vi "MoD Main-Optimize - HPLCv2 - Simulate.vi"() -> ()   [LabVIEW 2015]
uses:
  <vilib>/silver_ctls/ArrayMatrixCluster/Real Matrix NI_Silver.ctl
  <vilib>/addons/control/pid/pid.llb/PID Control Input Filter (DBL).vi
  <vilib>/addons/control/pid/autopid.llb/PID Online Autotuning (Relay Feedback).vi
  <vilib>/Analysis/Matrix/Numeric/Conversions/Array To Matrix - RA2.vi
  <vilib>/addons/control/pid/NI_PID_autopid.lvlib
  <vilib>/addons/control/pid/NI_PID_pid.lvlib
  <vilib>/Analysis/Matrix/NI_Matrix.lvlib
panel:
  out "running?":bool=TRUE
  out "new_reactor_volume":bool[](array[boolean])
  out "new_reactor_length":bool[](array[boolean])
  out "Phase_Sensor_voltage":dbl
  out "P_tot":dbl
  out "pause for ms":bool=TRUE
  out "stop_xl_write":bool=TRUE
  out "Num_exp_till_pause":i32
  out "Syringe_pump?":bool=TRUE
  out "System Error":bool=TRUE
  out "error out":errorcluster
  out "Pump setpoint(ul/min) 6":dbl format="%#_13g"
  out "Pump setpoint(ul/min) 5":dbl format="%#_13g"
  out "Pump setpoint(ul/min) 4":dbl format="%#_13g"
  out "Pump setpoint(ul/min) 3":dbl format="%#_13g"
  out "Pump setpoint(ul/min) 2":dbl format="%#_13g"
  out "Pump setpoint(ul/min) 1":dbl format="%#_13g"
  out "Volume (ul) 5":dbl format="%#_13g"
  out "Volume (ul) 4":dbl format="%#_13g"
  out "Volume (ul) 3":dbl format="%#_13g"
  out "Volume (ul) 2":dbl format="%#_13g"
  out "Volume (ul) 1":dbl format="%#_13g"
  in  "tau 5":dbl format="%#_13g"
  out "tau 4":dbl format="%#_13g"
  out "tau 3":dbl format="%#_13g"
  out "tau 2":dbl format="%#_13g"
  out "tau 1":dbl format="%#_13g"
  out "Reactor Length":dbl format="%#_13g"
  out "Flowrate Sensor 2":dbl format="%#_13g"
  out "Flowrate Sensor 1":dbl format="%#_13g"
  out "Pressure 2":dbl format="%#_13g"
  out "Pressure 1":dbl format="%#_13g"
  out "Temperature Control 5":bool=TRUE
  out "Temperature Control 4":bool=TRUE
  out "Temperature Control 3":bool=TRUE
  out "Temperature Control 2":bool=TRUE
  out "Temperature Control 1":bool=TRUE
  out "Temperature SP 5":dbl format="%#_g'C"
  out "Temperature SP 4":dbl format="%#_g'C"
  out "Temperature SP 3":dbl format="%#_g'C"
  out "Temperature SP 2":dbl format="%#_g'C"
  out "Temperature SP 1":dbl format="%#_g'C"
  in  "Bay Temperature 5":dbl
  in  "SSR Duration 5":dbl
  in  "SSR Duration 4":dbl
  in  "SSR Duration 3":dbl
  in  "SSR Duration 2":dbl
  in  "SSR Duration 1":dbl
  in  "Total Product Amount":dbl=1.0 format="%#_gml"
  out "Setup Error":bool=TRUE
  out "Error Message":string
  out "ID CTR":i32
  in  "Tab Control":T1(tab)
  out "Reagent pic 5":picture
  in  "reagent name 5":string
  out "Reagent Pic 4":picture
  in  "reagent name 4":string="octane"
  out "Reagent Pic 3":picture
  in  "reagent  name 3":string="methane"
  in  "Product name":string="benzoic acid"
  in  "reagent name 1":string="hexanedione"
  out "Reagent Pic 1":picture
  in  "Vr5":dbl format="%#_guL"
  in  "Vr4":dbl format="%#_guL"
  in  "Vr3":dbl format="%#_guL"
  in  "Vr2":dbl format="%#_guL"
  in  "Vr1":dbl format="%#_guL"
  in  "System decide help Button":bool
  in  "Reaction Scheme Confirm":bool
  in  "Synthesis Route Array":string[][](array[string])=[["hexanedione", ".5", "PhB(OH)2", "", "", ""], ["ethanol", ".5", "-", "-", "-", "-"], ["methane", ".1", "-", "-", "-", "-"], ["octane", ".1", "-", "-", "-", "-"]]
  in  "System decide help Button 2":bool
  out "Setup Confirm":bool=TRUE
  in  "BAY 1":u16(ring) items=["               Bypass", "         Heated Reactor", "    Small Heated Reator", "         Cooled Reactor", "      Packed Bed Reactor", "          Photo Reactor", "             Separator"]
  in  "BAY 5":u16(ring) items=["               Bypass", "         Heated Reactor", "    Small Heated Reactor", "         Cooled Reactor", "     Packed Bed Reactor", "         Photo Reactor", "             Separator"]
  in  "BAY 4":u16(ring)=1 items=["                Bypass", "         Heated Reactor", "    Small Heated Reactor", "         Cooled Reactor", "     Packed Bed Reactor", "         Photo Reactor", "             Separator"]
  in  "BAY 3":u16(ring) items=["               Bypass", "         Heated Reactor", "    Small Heated Reactor", "         Cooled Reactor", "     Packed Bed Reactor", "          Photo Reactor", "             Separator"]
  in  "BAY 2":u16(ring)=1 items=["               Bypass", "         Heated Reactor", "    Small Heated Reactor", "         Cooled Reactor", "      Packed Bed Reactor", "          Photo Reactor", "             Separator"]
  out "Reagent Pic 2":picture
  out "Product Pic":picture
  in  "reagent name 2":string="ethanol"
  in  "reagent name 6":string
  out "Reagent Pic 6":picture
  in  "System Parameters Help Button":bool
  out "Setup Confirm 2":bool
  in  "System Parameters Confirm Button":bool
  in  "Bay Parameters":T2={"Bay 1 "={"Pump 1 Flowrate"=0.0, "optimize_temp"=FALSE, "optimize_tau"=FALSE, "Run at set flowrate"=FALSE, "Pump 2 Flowrate"=0.0, "Temperature Params"=[40.0, 100.0, 100.0], "pump params 1"=[32.0, 325.0, 325.0], "pump params 2"=[32.0, 325.0, 325.0], "Temperature"=0.0, "Run at set temperature"=FALSE}, "Bay 2 "={"Pump 3 Flowrate"=0.0, "optimize_temp"=TRUE, "optimize_tau"=TRUE, "Run at set flowrate"=FALSE, "Temperature Params"=[40.0, 100.0, 100.0], "Resisdence time params"=[65.0, 650.0, 650.0], "pump_at_ratio"=FALSE, "pump_num_ratio"=0.0, "Temperature"=0.0, "Run at set temperature"=FALSE}, "Bay 3 "={"Pump 4 Flowrate"=100.0, "optimize_temp"=FALSE, "optimize_tau"=FALSE, "Run at set flowrate"=TRUE, "Temperature Params"=[40.0, 100.0, 100.0], "Resisdence time params"=[0.0, 0.0, 0.0], "pump_at_ratio"=FALSE, "pump_num_ratio"=0.0, "Temperature "=0.0, "Run at set temperature"=FALSE}, "Bay 4 "={"Pump 5 Flowrate"=40.0, "Run at set flowrate"=FALSE, "optimize_temp"=TRUE, "optimize_tau"=FALSE, "Resisdence time params"=[0.0, 36.0, 225.0], "Temperature Params"=[40.0, 80.0, 80.0], "pump_at_ratio"=FALSE, "pump_num_ratio"=0.0, "Temperature"=0.0, "Run at set temperature"=FALSE}, "Bay 5 "={"Pump 6 Flowrate"=0.0, "Run at set flowrate"=FALSE, "optimize_temp"=FALSE, "optimize_tau"=FALSE, "Resisdence time params"=[0.0, 0.0, 0.0], "Temperature Params"=[0.0, 0.0, 0.0], "pump_at_ratio"=FALSE, "pump_num_ratio"=0.2, "Temperature"=0.0, "Run at set temperature"=FALSE}, "Excel File Name"="C:\\Users\\Admin\\Dropbox (MIT)\\MoD Files\\Data\\simulations", "hplc File Name"="C:\\Users\\Admin\\Documents\\Data\\HPLC", "Matlab File"="C:\\Users\\Admin\\Dropbox (MIT)\\MoD Files\\Data\\simulation", "Syringe for Pump 2?"=FALSE, "Num_conditons_per_wait"=1.0, "Continue from previous optimization?"=FALSE, "Total Number of Experiments 2"=33.0, "Hplc Wait time(min)"=9.2, "increas_decrease_hplc_peak"=FALSE, "Internal Standard?"=FALSE, "ISTD start"=0.0, "ISTD end"=0.0, "hplc_start"=2.0, "hplc_end"=5.0, "throughput_yield"=FALSE} {"Hplc Wait time(min)" format="%#_13g"; "Bay 5"."Temperature Params" format="%#_g'C"; "Bay 4"."Temperature Params" format="%#_g'C"; "Bay 3"."Temperature Params" format="%#_g'C"; "Bay 2"."Temperature Params" format="%#_g'C"; "Bay 1"."Temperature Params" format="%#_g'C"}
  out "System Confirm Not Clicked":string
  out "best_exp_num":dbl=1.0
  out "temperature_best":dbl[](array[numeric])
  out "Flowrates(ul/min)_best":dbl[](array[numeric])
  out "System Status":u16(ring)=2 caption="Sy" items=["System  Error", "System Running", "System Standby"]
  out "Current Experiment":dbl=1.0
  out "Total Number of Experiments":dbl=33.0
  out "Phase Sensor Chart":T3(graph)
  out "HPLC Analysis":bool
  out "Equlibrating Temperature":bool
  out "Flushing System":bool
  out "Calculate condition":bool
  out "Temperature 5":dbl format="%#_g'C"
  out "Temperature 4":dbl format="%#_g'C"
  out "Temperature 3":dbl format="%#_g'C"
  out "Temperature 2":dbl format="%#_g'C"
  out "Temperature 1":dbl format="%#_g'C"
  out "Flowrate Chart":T4(graph)
  out "Teperature Chart":T5(graph)
  out "Pump Setpoints Chart":T5(graph)
  out "Pressure Chart":T5(graph)
  out "Optimization_loop_index":i32
  out "curr_wait_time":dbl
  out "total_flush_time":dbl
  out "Temp SS? 5":bool=TRUE
  out "Temp SS? 4":bool=TRUE
  out "Temp SS? 3":bool=TRUE
  out "Temp SS? 2":bool=TRUE
  out "Temp SS? 1":bool=TRUE
  out "System Flushed?":bool
  out "stop_button clicked":bool
  out "experiment history":T6
  in  "Number of System Flushes per condtion":dbl
  in  "calculate volume 3":bool
  in  "calculate volume 2":bool
  in  "calculate volume 1":bool
  in  "calculate volume 4":bool
  in  "calculate volume 5":bool
  in  "Extra system dead volume":dbl format="%#_gul"
  in  "new reactor length? 1":bool
  in  "tube_length(in)":dbl[](array[numeric])=[188.0, 188.0, 10.0, 10.0, 10.0]
  out "Pause Before Analysis":bool
  out "Chiller COMM Port":bool
  out "Arduino COMM Port 2":bool
  out "Temperature Sensor COMM Port":bool
  out "Flow Rate":bool
  out "Pressure":bool
  out "Pump COMM Port":bool
  in  "COMM Port :: Milligat Pumps":refnum<visa-resource-name>="COM10"
  in  "Arduino COMM Port":refnum<visa-resource-name>="COM3"
  in  "Sample Valve COMM::Port":refnum<visa-resource-name>="COM6"
  in  "COMM Port:: Harvard Syringe Pump":refnum<visa-resource-name>="COM5"
  in  "tube_id(in)":enum16{".01", ".02", ".03", ".04"}[](array[ring])=[enum.".02", enum.".03", enum.".03", enum.".03", enum.".03"]
  out "Total System Resisdence Time(min)":dbl
  in  "Debug_run_button":bool
  in  "new reactor length? 2":bool
  in  "new reactor length? 3":bool
  in  "new reactor length? 4":bool
  in  "new reactor length? 5":bool
  out "Stop":bool=TRUE
  in  "Run_Stop_cluster":T7
  # "Molecules on Demand"
  # "Synthetic Route"
  # "5"
  # "6"
  # "4"
  # "Product"
  # "1"
  # "2"
  # "3"
  # "Reagent List"
  # "Concentration(M)"
  # "Molecule"
  # "1"
  # "1"
  # "2"
  # "2"
  # "3"
  # "3"
  # "4"
  # "4"
  # "5"
  # "6"
  # "5"
  # "6"
  # "Product"
  # "Reactor Volume:"
  # "Optimization Parameters"
  # "Pause after"
  # "Experiments"
  # "Optimize for"
  # "to"
  # "of HPLC Peak from"
  # "from"
  # "to"
  # "min"
  # "min"
  # "HPLC runtime"
  # "# Iterations"
  # "Reporting"
  # "Excel Output File Name"
  # "HPLC File Path"
  # "MATLAB File Path"
  # "Temperature"
  # "Flowrate(ul/min)"
  # "Lower Bound"
  # "Upper Bound"
  # "Optimize?"
  # "-or-"
  # "Run at"
  # "times incoming flow"
  # "Setpoint"
  # "Temperature"
  # "Flowrate(ul/min)"
  # "Lower Bound"
  # "Upper Bound"
  # "Optimize?"
  # "-or-"
  # "Run at"
  # "times incoming flow"
  # "Setpoint"
  # "Temperature"
  # "Flowrate(ul/min)"
  # "Lower Bound"
  # "Upper Bound"
  # "Optimize?"
  # "-or-"
  # "Run at"
  # "times incoming flow"
  # "Setpoint"
  # "Temperature"
  # "Flowrate 3 (ul/min)"
  # "Lower Bound"
  # "Upper Bound"
  # "Optimize?"
  # "-or-"
  # "Run at"
  # "times incoming flow"
  # "Setpoint"
  # "Temperature"
  # "Flowrate 1(ul/min)"
  # "Flowrate 2(ul/min)"
  # "Lower Bound"
  # "Upper Bound"
  # "Optimize?"
  # "Setpoint"
  # "Pressure (psi)"
  # "System Status"
  # "Temperature('C)"
  # "BAY"
  # "1"
  # "2"
  # "3"
  # "4"
  # "5"
  # "Pump Flowrate Setpoint(ul/min)"
  # "Flowrate (ul/min)"
  # "Phase Sensor"
  # "Current Experiment"
  # "Temperature('C)"
  # "Flowrate(ul/min)"
  # "Exp"
  # "Current Best Condition"
  # "Time to reach steady state:"
  # "Current Wait Time:"
  # "Experimental Steps"
  # "Calculated new conditions"
  # "Flushed System"
  # "Analyzed HPLC"
  # "Equilibrated Temperature"
  # "Tube Length (cm)"
  # "Bay"
  # "Tube ID (in)"
  # "Calculate Volume"
  # "Use new tube length"
  # "1."
  # "2."
  # "3."
  # "4."
  # "5."
  # "Reactor Lengths\n*Heated Reactor - 188cm * Small Reactor - 99cm * Bypass - 10cm * Separator - *"
  # "All Experimental Data"
  # "P1"
  # "P2"
  # "P3"
  # "P4"
  # "P5"
  # "P6"
  # "T1"
  # "T2"
  # "T3"
  # "T4"
  # "T5"
  # "Obj_fun"
  # "HPLC_Data"
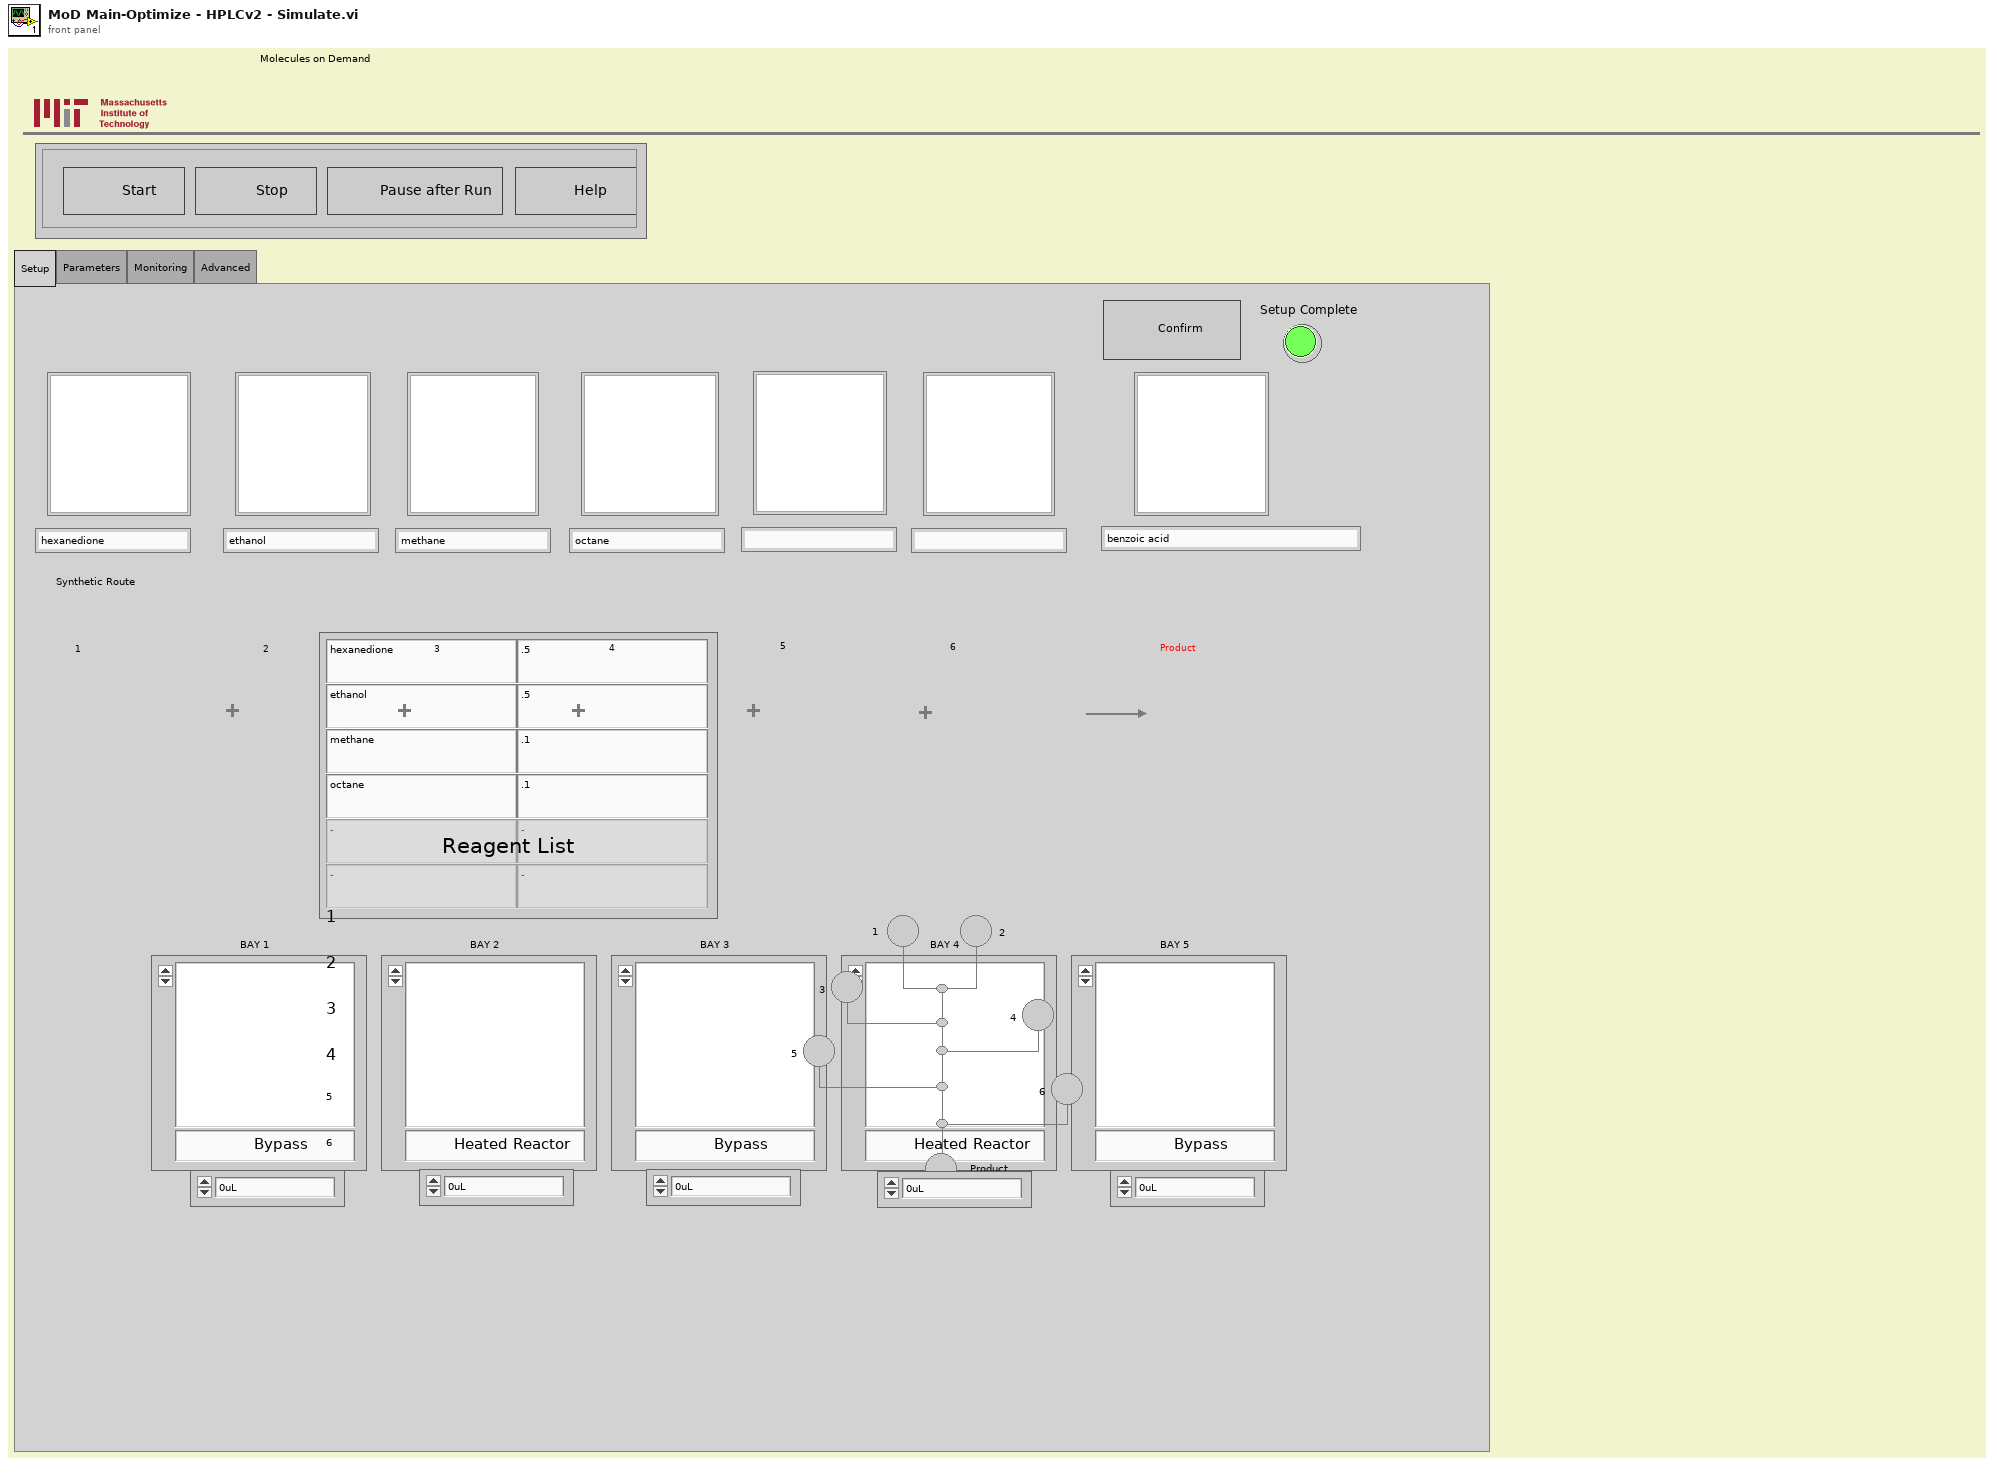
[diagram p1: front panel]
types:
  T1 = enum32{"Setup", "Parameters", "Monitoring", "Advanced"}
  T2 = cluster{"Bay 1 ":cluster{"Pump 1 Flowrate":dbl, "optimize_temp":bool, "optimize_tau":bool, "Run at set flowrate":bool, "Pump 2 Flowrate":dbl, "Temperature Params":dbl[], "pump params 1":dbl[], "pump params 2":dbl[], "Temperature":dbl, "Run at set temperature":bool}, "Bay 2 ":cluster{"Pump 3 Flowrate":dbl, "optimize_temp":bool, "optimize_tau":bool, "Run at set flowrate":bool, "Temperature Params":dbl[], "Resisdence time params":dbl[], "pump_at_ratio":bool, "pump_num_ratio":dbl, "Temperature":dbl, "Run at set temperature":bool}, "Bay 3 ":cluster{"Pump 4 Flowrate":dbl, "optimize_temp":bool, "optimize_tau":bool, "Run at set flowrate":bool, "Temperature Params":dbl[], "Resisdence time params":dbl[], "pump_at_ratio":bool, "pump_num_ratio":dbl, "Temperature ":dbl, "Run at set temperature":bool}, "Bay 4 ":cluster{"Pump 5 Flowrate":dbl, "Run at set flowrate":bool, "optimize_temp":bool, "optimize_tau":bool, "Resisdence time params":dbl[], "Temperature Params":dbl[], "pump_at_ratio":bool, "pump_num_ratio":dbl, "Temperature":dbl, "Run at set temperature":bool}, "Bay 5 ":cluster{"Pump 6 Flowrate":dbl, "Run at set flowrate":bool, "optimize_temp":bool, "optimize_tau":bool, "Resisdence time params":dbl[], "Temperature Params":dbl[], "pump_at_ratio":bool, "pump_num_ratio":dbl, "Temperature":dbl, "Run at set temperature":bool}, "Excel File Name":string, "hplc File Name":string, "Matlab File":string, "Syringe for Pump 2?":bool, "Num_conditons_per_wait":dbl, "Continue from previous optimization?":bool, "Total Number of Experiments 2":dbl, "Hplc Wait time(min)":dbl, "increas_decrease_hplc_peak":bool, "Internal Standard?":bool, "ISTD start":dbl, "ISTD end":dbl, "hplc_start":dbl, "hplc_end":dbl, "throughput_yield":bool}
  T3 = cluster{"[0]":u8, "[1]":u8, "[2]":u8, "[3]":u8, "[4]":u8, "[5]":u8, "[6]":u8, "[7]":u8, "[8]":u8}
  T4 = cluster{"[0]":i32, "[1]":i32, "[2]":i32, "[3]":i32, "[4]":i32, "[5]":i32, "[6]":i32, "[7]":i32, "[8]":i32}
  T5 = cluster{"[0]":dbl, "[1]":dbl, "[2]":dbl, "[3]":dbl, "[4]":dbl, "[5]":dbl, "[6]":dbl, "[7]":dbl, "[8]":dbl}
  T6 = typedef "Real Matrix NI_Silver.ctl" = dbl[][]
  T7 = cluster{"Stop":bool, "Run":bool, "Stop Run Button":bool, "Help Button":bool}
  T8 = cluster{"Proportional gain Kc":dbl, "Integral time Ti (sec)":dbl, "Derivative time Ti (sec)":dbl}
  T9 = cluster{"type of controller":enum16{"P", "PI", "PID"}, "relay cycles":i32, "relay amplitude":dbl, "control specifications":enum16{"Fast", "Normal", "Slow"}, "PV noise level":dbl}
  T10 = typedef "imagedata.ctl" = cluster{"image type":i32, "image depth":i32, "image":u8[], "mask":u8[], "colors":u32[], "Rectangle":cluster{"left":i16, "top":i16, "right":i16, "bottom":i16}}
  T11 = cluster{"proportional gain (Kc)":dbl, "integral time (Ti, min)":dbl, "derivative time (Td, min)":dbl}
  T12 = enum16{"Left Button", "Center Button", "Right Button", "Window Close"}
  T13 = typedef "NI_Matrix.lvlib/RealMatrix.ctl" = dbl[][]
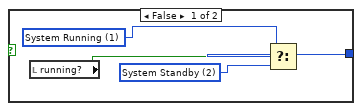
[diagram p4: hidden frame]
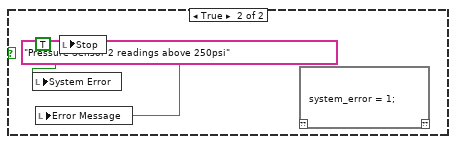
[diagram p5: hidden frame]
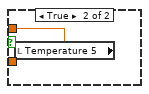
[diagram p7: hidden frame]
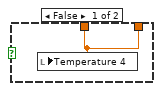
[diagram p8: hidden frame]
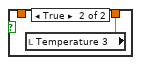
[diagram p9: hidden frame]
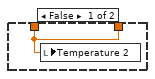
[diagram p10: hidden frame]
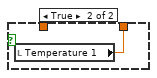
[diagram p11: hidden frame]
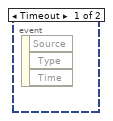
[diagram p12: hidden frame]
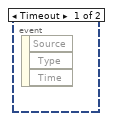
[diagram p14: hidden frame]
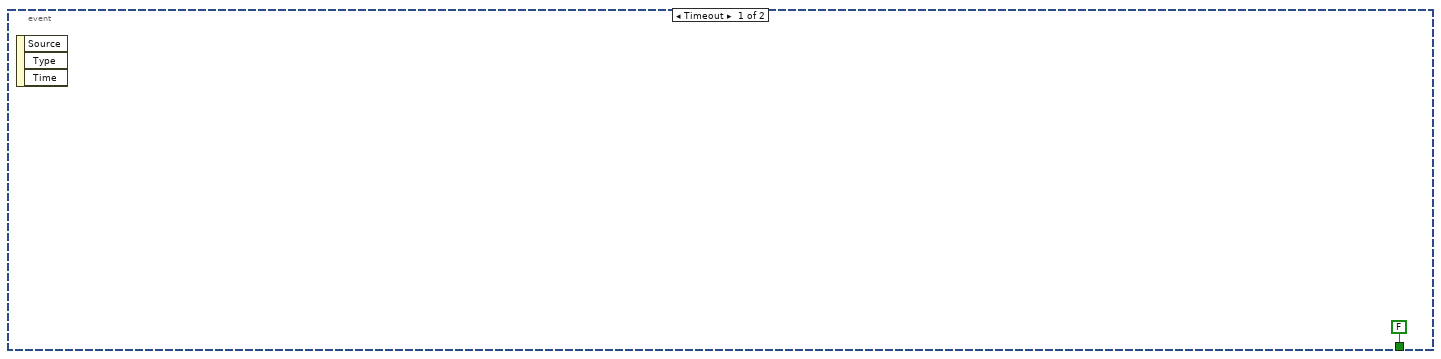
[diagram p17: hidden frame]
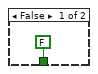
[diagram p18: hidden frame]
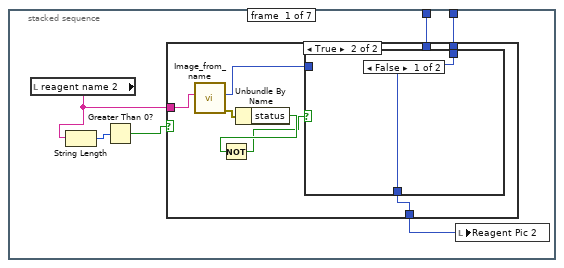
[diagram p19: hidden frame]
diagram:
  # "Assume User always uses the first bay first"
  n1 = flat-sequence {
    tunnel: ["COMM Port :: Milligat Pumps"] -> w6
    tunnel: ["Arduino COMM Port"] -> w5
    tunnel: ["COMM Port:: Harvard Syringe Pump"] -> w2
    tunnel: ["Bay Parameters"] -> w1
    tunnel: [w54] -> w7
    tunnel: w6 -> [w54]
    tunnel: w5 -> [_]
    tunnel: [w48] -> w4
    tunnel: [w46] -> w3
    tunnel: w2 -> [w46]
    tunnel: w1 -> [w44]
    tunnel: w7 -> [w58]
    tunnel: w4 -> [w57]
    tunnel: w3 -> [w55]
    frame #0 {
      w32 = FALSE ("Equlibrating Temperature")
      n2 = disable-structure shown="Disabled" {
        frame Disabled {
          # "IR Sensor"
        }
        frame Enabled {
        }
      }
      n3 = script code="TempArr1=[23 23 23 23 23 23 23 23 23 23]';\nTempArr2=[23 23 23 23 23 23 23 23 23 23]';\nTempArr3=[23 23 23 23 23 23 23 23 23 23]';\nTempArr4=[23 23 23 23 23 23 23 23 23 23]';\nTempArr5=[23 23 23 23 23 23 23 23 23 23]';\ntemp_error1 =0;\ntemp_error2 =0;\ntemp_error3 =0;\ntemp_error4 =0;\ntemp_error5 =0;\ntemp_check1 = 0;\ntemp_check2 = 0;\ntemp_check3 = 0;\ntemp_check4 = 0;\ntemp_check5 = 0;\nT1=23;\nT2=23;\nT3=23;\nT4=23;\nT5=23;"() -> ()  [unwired: 1 in, 1 out]
      n4 = Build Array("calculate volume 1", "calculate volume 2", "calculate volume 3", "calculate volume 4", "calculate volume 5") -> (→"new_reactor_volume":bool[])
      n5 = Build Array("new reactor length? 1", "new reactor length? 2", "new reactor length? 3", "new reactor length? 4", "new reactor length? 5") -> (→"new_reactor_length":bool[])
      "Stop" <- FALSE ("Stop")
      "ID CTR" <- 0
      "Setup Confirm" <- FALSE ("Setup Confirm")
      "Error Message" <- "System shutdown sucessfully. No errors to report." ("Error Message")
      "Setup Error" <- FALSE ("Setup Error")
      "Reactor Length" <- 10.5
      "System Error" <- FALSE ("System Error")
      "Num_exp_till_pause" <- 0 ("Num_exp_till_pause")
      "Equlibrating Temperature" <- w32
      "Calculate condition" <- w32
      "Flushing System" <- w32
      "HPLC Analysis" <- w32
      "stop_xl_write" <- FALSE ("stop_xl_write")
      "Pump setpoint(ul/min) 1" <- 0.0 ("Pump setpoint(ul/min) 1")
      "Pump setpoint(ul/min) 2" <- 0.0 ("Pump setpoint(ul/min) 2")
      "Pump setpoint(ul/min) 4" <- 0.0 ("Pump setpoint(ul/min) 4")
      "Pump setpoint(ul/min) 6" <- 0.0 ("Pump setpoint(ul/min) 6")
      "Pump setpoint(ul/min) 3" <- 0.0 ("Pump setpoint(ul/min) 3")
      "Pump setpoint(ul/min) 5" <- 0.0 ("Pump setpoint(ul/min) 5")
      "pause for ms" <- FALSE ("pause for ms")
      "Setup Confirm 2" <- FALSE ("Setup Confirm 2")
      "running?" <- FALSE ("running?")
    }
    frame #1 {
      w43 = FALSE
      w53 = 23
      (unwired) path "C:/Users/User1/Documents/Lab/MoD/Images"
      n6 = disable-structure shown="Disabled" {
        frame Disabled {
          n7 = local read "BAY 2"() -> ()  [unwired: 1 out]
          n8 = local read "BAY 3"() -> ()  [unwired: 1 out]
          n9 = local read "BAY 4"() -> ()  [unwired: 1 out]
          n10 = local read "BAY 5"() -> ()  [unwired: 1 out]
          n11 = local read "BAY 1"() -> ()  [unwired: 1 out]
        }
        frame Enabled {
        }
      }
      n12 = local write "Debug_run_button"(TRUE) -> ()
      n13 = local write "System Parameters Confirm Button"(w43) -> ()
      n14 = local write "Setup Confirm 2"(w43) -> ()
      n15 = Unbundle By Name(w44) -> ("Syringe for Pump 2?"=→"Syringe_pump?":bool)
      n16 = local write "Temperature 1"(w53) -> ()
      n17 = local write "Temperature 2"(w53) -> ()
      n18 = local write "Temperature 3"(w53) -> ()
      n19 = local write "Temperature 4"(w53) -> ()
      n20 = local write "Temperature 5"(w53) -> ()
      n21 = local write "Temperature SP 1"(w53) -> ()
      n22 = local write "Temperature SP 2"(w53) -> ()
      n23 = local write "Temperature SP 3"(w53) -> ()
      n24 = local write "Temperature SP 4"(w53) -> ()
      n25 = local write "Temperature SP 5"(w53) -> ()
      n26 = Current VI's Path() -> (path=w52:path)
      n27 = Strip Path(path=w52) -> (stripped path=w50:path)  [unwired: 1 out]
      n28 = Strip Path(path=w50) -> (stripped path=w49:path)  [unwired: 1 out]
      n29 = Build Path(base path=w49, name or relative path="MATLAB") -> (appended path=w48:path)
    }
    frame #2 {
      # "Main Help Dialog Popup"
      n30 = while {
        stop <- w1172 stop-if-true
        n31 = event shown="[6] \"Run_Stop_cluster.Run\": Value Change" {
          selector: _ -> [_ _ _ _ _ _ _]
          dyn-events: _ -> [_ _ _ _ _ _ _]
          timeout: 100 -> [_ _ _ _ _ _ _]
          event Timeout {
            n32 = event-data() -> ()  [unwired: 1 in, 3 out]
          }
          event "Run_Stop_cluster.Help Button": Value Change {
            n33 = local read "Run_Stop_cluster"() -> (w1175:T7)
            n34 = event-data() -> ()  [unwired: 1 in, 4 out]
            n35 = Unbundle By Name(w1175) -> ("Help Button"=w1174:bool)
            n36 = case shown="True" w1174 {
              frame False {
              }
              frame True {
                n37 = call "help.vi"() -> ()  [unwired: 11 in]
              }
            }
          }
          event "System decide help Button": Value Change {
            n38 = event-data() -> ()  [unwired: 1 in, 5 out]
            n39 = call "help_synthesis_man-auto_instructions.vi"() -> ()  [unwired: 12 in]
          }
          event "System Parameters Help Button": Value Change {
            n40 = event-data() -> ()  [unwired: 1 in, 5 out]
            n41 = call "help_parameters_setup.vi"() -> ()  [unwired: 12 in]
          }
          event "System decide help Button 2": Value Change {
            n42 = event-data() -> ()  [unwired: 1 in, 5 out]
            n43 = call "help_synthesis_route_instructions.vi"() -> ()  [unwired: 12 in]
          }
          event "Run_Stop_cluster.Stop": Value Change {
            n44 = event-data() -> ()  [unwired: 1 in, 5 out]
            n45 = local write "Stop"(TRUE) -> ()
          }
          event "Run_Stop_cluster.Run": Value Change {
            n46 = event-data() -> ()  [unwired: 1 in, 5 out]
            n47 = local write "running?"(TRUE) -> ()
          }
        }
        n48 = local read "Stop"() -> (w1172:bool)
      }
      n49 = stacked-sequence {
        tunnel: w58 -> [_ _ _ _]
        tunnel: w57 -> [_ w364 _ _]
        tunnel: w55 -> [_ _ _ w526]
        frame #0 {
          # "System Setup"
          n50 = while {
            stop <- w160 stop-if-true
            n51 = event shown="[1] \"Reaction Scheme Confirm\": Value Change" {
              selector: _ -> [_ _]
              dyn-events: _ -> [_ _]
              timeout: 400 -> [_ _]
              tunnel: [FALSE w180] -> w162
              event Timeout {
                n52 = event-data() -> ()  [unwired: 1 in, 3 out]
              }
              event "Reaction Scheme Confirm": Value Change {
                n53 = event-data() -> ()  [unwired: 1 in, 6 out]
                n54 = local read "Reaction Scheme Confirm"() -> (w184:bool)
                n55 = local read "Setup Confirm"() -> (w182:bool)
                n56 = Not(x=w182) -> (.not. x?=w181:bool)
                n57 = And(x=w184, y=w181) -> (x .and. y?=w183:bool)
                n58 = case shown="True" w183 {
                  tunnel: [FALSE w186] -> w180
                  frame False {
                  }
                  frame True {
                    n59 = flat-sequence {
                      tunnel: [w354] -> w186
                      frame #0 {
                        n60 = local write "Setup Error"(FALSE) -> ()
                      }
                      frame #1 {
                        n61 = local read "Synthesis Route Array"() -> (w190:string[][])
                        n62 = Index Array(array=w190, index (col)=0 ("disabled index (col)")) -> (element=w188:string[])  [unwired: 1 in]
                        n63 = Array Size(array=w188) -> (size(s)=w191:i32)
                        n64 = script code="MATLAB script"("reagentNum"=w191) -> ()  [unwired: 1 in, 1 out]
                      }
                      frame #2 {
                        w194 = "C:\\Users\\HPLC\\Dropbox (MIT)\\MoD Files\\LabVIEW\\Mod 2014\\MoD Main Folder\\Chemical Image\\" ("string")
                        n65 = String To Path(string=w194) -> (path=w200:path)
                        n66 = Build Path(base path=w200, name or relative path="image_not_found3.jpg") -> (appended path=w199:path)
                        n67 = String To Path(string=w194) -> (path=w197:path)
                        n68 = call <vilib>:"Read JPEG File.vi"("path to JPEG file"=w199) -> ("image data"=w202:T10)  [unwired: 1 in, 9 out]
                        n69 = Build Path(base path=w197, name or relative path="blank image.jpg") -> (appended path=w195:path)
                        n70 = call <vilib>:"Read JPEG File.vi"("path to JPEG file"=w195) -> ("image data"=w198:T10)  [unwired: 1 in, 9 out]
                        n71 = call <vilib>:"Draw Flattened Pixmap.vi"("image data"=w202) -> ("new picture"=w193:picture)  [unwired: 3 in, 5 out]
                        n72 = call <vilib>:"Draw Flattened Pixmap.vi"("image data"=w198) -> ("new picture"=w192:picture)  [unwired: 3 in, 5 out]
                        n73 = stacked-sequence {
                          tunnel: w193 -> [w208 w225 w242 w259 w276 w290 w307]
                          tunnel: w192 -> [w206 w223 w240 w257 w274 w291 w308]
                          frame #0 {
                            n74 = local read "reagent name 2"() -> (w204:string)
                            n75 = String Length(string=w204) -> (length=w207:i32)
                            n76 = Greater Than 0?(x=w207) -> (x > 0?=w205:bool)
                            n77 = case shown="True" w205 {
                              tunnel: w208 -> [_ w214]
                              tunnel: w206 -> [w209 _]
                              tunnel: [w209 w213] -> w203
                              tunnel: w204 -> [_ w212]
                              frame False {
                              }
                              frame True {
                                n78 = call "Image_from_name.vi"("Chemical Name"=w212) -> ("error out"=w215:errorcluster, "Downloaded Picture"=w216:picture)  [unwired: 8 in, 1 out]
                                n79 = Unbundle By Name(w215) -> ("status"=w211:bool)
                                n80 = Not(x=w211) -> (.not. x?=w210:bool)
                                n81 = case shown="False" w210 {
                                tunnel: w216 -> [_ w219]
                                tunnel: [w217 w218] -> w213
                                tunnel: w214 -> [w217 _]
                                frame False {
                                }
                                frame True {
                                n82 = call <vilib>:"Draw Flattened Pixmap.vi"("picture"=w219) -> ("new picture"=w218:picture)  [unwired: 8 in]
                                }
                                }
                              }
                            }
                            n83 = local write "Reagent Pic 2"(w203) -> ()
                          }
                          frame #1 {
                            n84 = local read "reagent name 1"() -> (w220:string)
                            n85 = String Length(string=w220) -> (length=w224:i32)
                            n86 = Greater Than 0?(x=w224) -> (x > 0?=w222:bool)
                            n87 = case shown="True" w222 {
                              tunnel: w225 -> [_ w231]
                              tunnel: w223 -> [w226 _]
                              tunnel: [w226 w230] -> w221
                              tunnel: w220 -> [_ w229]
                              frame False {
                              }
                              frame True {
                                n88 = call "Image_from_name.vi"("Chemical Name"=w229) -> ("error out"=w232:errorcluster, "Downloaded Picture"=w233:picture)  [unwired: 8 in, 1 out]
                                n89 = Unbundle By Name(w232) -> ("status"=w228:bool)
                                n90 = Not(x=w228) -> (.not. x?=w227:bool)
                                n91 = case shown="True" w227 {
                                tunnel: w233 -> [_ w236]
                                tunnel: [w234 w235] -> w230
                                tunnel: w231 -> [w234 _]
                                frame False {
                                }
                                frame True {
                                n92 = call <vilib>:"Draw Flattened Pixmap.vi"("picture"=w236) -> ("new picture"=w235:picture)  [unwired: 8 in]
                                }
                                }
                              }
                            }
                            n93 = local write "Reagent Pic 1"(w221) -> ()
                          }
                          frame #2 {
                            n94 = local read "Product name"() -> (w237:string)
                            n95 = String Length(string=w237) -> (length=w241:i32)
                            n96 = Greater Than 0?(x=w241) -> (x > 0?=w239:bool)
                            n97 = case shown="True" w239 {
                              tunnel: w242 -> [_ w248]
                              tunnel: w240 -> [w243 _]
                              tunnel: [w243 w247] -> w238
                              tunnel: w237 -> [_ w246]
                              frame False {
                              }
                              frame True {
                                n98 = call "Image_from_name.vi"("Chemical Name"=w246) -> ("error out"=w249:errorcluster, "Downloaded Picture"=w250:picture)  [unwired: 8 in, 1 out]
                                n99 = Unbundle By Name(w249) -> ("status"=w244:bool)
                                n100 = Not(x=w244) -> (.not. x?=w245:bool)
                                n101 = case shown="False" w245 {
                                tunnel: w250 -> [_ w253]
                                tunnel: [w251 w252] -> w247
                                tunnel: w248 -> [w251 _]
                                frame False {
                                }
                                frame True {
                                n102 = call <vilib>:"Draw Flattened Pixmap.vi"("picture"=w253) -> ("new picture"=w252:picture)  [unwired: 8 in]
                                }
                                }
                              }
                            }
                            n103 = local write "Product Pic"(w238) -> ()
                          }
                          frame #3 {
                            n104 = local read "reagent name 6"() -> (w254:string)
                            n105 = String Length(string=w254) -> (length=w258:i32)
                            n106 = Greater Than 0?(x=w258) -> (x > 0?=w256:bool)
                            n107 = case shown="True" w256 {
                              tunnel: w259 -> [_ w265]
                              tunnel: w257 -> [w260 _]
                              tunnel: [w260 w264] -> w255
                              tunnel: w254 -> [_ w263]
                              frame False {
                              }
                              frame True {
                                n108 = call "Image_from_name.vi"("Chemical Name"=w263) -> ("error out"=w266:errorcluster, "Downloaded Picture"=w267:picture)  [unwired: 8 in, 1 out]
                                n109 = Unbundle By Name(w266) -> ("status"=w261:bool)
                                n110 = Not(x=w261) -> (.not. x?=w262:bool)
                                n111 = case shown="False" w262 {
                                tunnel: w267 -> [_ w270]
                                tunnel: [w268 w269] -> w264
                                tunnel: w265 -> [w268 _]
                                frame False {
                                }
                                frame True {
                                n112 = call <vilib>:"Draw Flattened Pixmap.vi"("picture"=w270) -> ("new picture"=w269:picture)  [unwired: 8 in]
                                }
                                }
                              }
                            }
                            n113 = local write "Reagent Pic 6"(w255) -> ()
                          }
                          frame #4 {
                            n114 = local read "reagent name 5"() -> (w271:string)
                            n115 = String Length(string=w271) -> (length=w275:i32)
                            n116 = Greater Than 0?(x=w275) -> (x > 0?=w273:bool)
                            n117 = case shown="True" w273 {
                              tunnel: w276 -> [_ w282]
                              tunnel: w274 -> [w277 _]
                              tunnel: [w277 w281] -> w272
                              tunnel: w271 -> [_ w280]
                              frame False {
                              }
                              frame True {
                                n118 = call "Image_from_name.vi"("Chemical Name"=w280) -> ("error out"=w283:errorcluster, "Downloaded Picture"=w284:picture)  [unwired: 8 in, 1 out]
                                n119 = Unbundle By Name(w283) -> ("status"=w278:bool)
                                n120 = Not(x=w278) -> (.not. x?=w279:bool)
                                n121 = case shown="False" w279 {
                                tunnel: w284 -> [_ w287]
                                tunnel: [w285 w286] -> w281
                                tunnel: w282 -> [w285 _]
                                frame False {
                                }
                                frame True {
                                n122 = call <vilib>:"Draw Flattened Pixmap.vi"("picture"=w287) -> ("new picture"=w286:picture)  [unwired: 8 in]
                                }
                                }
                              }
                            }
                            n123 = local write "Reagent pic 5"(w272) -> ()
                          }
                          frame #5 {
                            n124 = local read "reagent name 4"() -> (w288:string)
                            n125 = String Length(string=w288) -> (length=w293:i32)
                            n126 = Greater Than 0?(x=w293) -> (x > 0?=w292:bool)
                            n127 = case shown="True" w292 {
                              tunnel: w290 -> [_ w299]
                              tunnel: w291 -> [w294 _]
                              tunnel: [w294 w298] -> w289
                              tunnel: w288 -> [_ w297]
                              frame False {
                              }
                              frame True {
                                n128 = call "Image_from_name.vi"("Chemical Name"=w297) -> ("error out"=w300:errorcluster, "Downloaded Picture"=w301:picture)  [unwired: 8 in, 1 out]
                                n129 = Unbundle By Name(w300) -> ("status"=w295:bool)
                                n130 = Not(x=w295) -> (.not. x?=w296:bool)
                                n131 = case shown="False" w296 {
                                tunnel: w301 -> [_ w304]
                                tunnel: [w302 w303] -> w298
                                tunnel: w299 -> [w302 _]
                                frame False {
                                }
                                frame True {
                                n132 = call <vilib>:"Draw Flattened Pixmap.vi"("picture"=w304) -> ("new picture"=w303:picture)  [unwired: 8 in]
                                }
                                }
                              }
                            }
                            n133 = local write "Reagent Pic 4"(w289) -> ()
                          }
                          frame #6 {
                            n134 = local read "reagent  name 3"() -> (w305:string)
                            n135 = String Length(string=w305) -> (length=w310:i32)
                            n136 = Greater Than 0?(x=w310) -> (x > 0?=w309:bool)
                            n137 = case shown="True" w309 {
                              tunnel: w307 -> [_ w316]
                              tunnel: w308 -> [w311 _]
                              tunnel: [w311 w315] -> w306
                              tunnel: w305 -> [_ w314]
                              frame False {
                              }
                              frame True {
                                n138 = call "Image_from_name.vi"("Chemical Name"=w314) -> ("error out"=w317:errorcluster, "Downloaded Picture"=w318:picture)  [unwired: 8 in, 1 out]
                                n139 = Unbundle By Name(w317) -> ("status"=w312:bool)
                                n140 = Not(x=w312) -> (.not. x?=w313:bool)
                                n141 = case shown="False" w313 {
                                tunnel: w318 -> [_ w321]
                                tunnel: [w319 w320] -> w315
                                tunnel: w316 -> [w319 _]
                                frame False {
                                }
                                frame True {
                                n142 = call <vilib>:"Draw Flattened Pixmap.vi"("picture"=w321) -> ("new picture"=w320:picture)  [unwired: 8 in]
                                }
                                }
                              }
                            }
                            n143 = local write "Reagent Pic 3"(w306) -> ()
                          }
                        }
                      }
                      frame #3 {
                        n144 = local read "BAY 1"() -> (w332:u16)
                        n145 = local read "BAY 2"() -> (w331:u16)
                        n146 = local read "BAY 3"() -> (w330:u16)
                        n147 = local read "BAY 4"() -> (w329:u16)
                        n148 = local read "BAY 5"() -> (w328:u16)
                        n149 = local read "tube_id(in)"() -> (w339:enum16{".01", ".02", ".03", ".04"}[])
                        n150 = local read "Vr4"() -> (w342:dbl)
                        n151 = local read "tube_length(in)"() -> (w340:dbl[])
                        n152 = Build Array(w332, w331, w330, w329, w328) -> (w327:u16[])
                        n153 = local read "Vr3"() -> (w343:dbl)
                        n154 = local read "new_reactor_length"() -> (w337:bool[])
                        n155 = local read "Vr1"() -> (w345:dbl)
                        n156 = local read "Vr5"() -> (w341:dbl)
                        n157 = local read "Vr2"() -> (w344:dbl)
                        n158 = local read "new_reactor_volume"() -> (w335:bool[])
                        n159 = for {
                          N: 5 -> [_]
                          tunnel: w335 -> [w349] mode=indexing
                          tunnel: [w346] -> w333 mode=indexing
                          n160 = Select(t=1.0, s=w349, f=0.0) -> (s? t:f=w346:dbl)
                        }
                        n161 = for {
                          N: 5 -> [_]
                          tunnel: w337 -> [w353] mode=indexing
                          tunnel: [w350] -> w336 mode=indexing
                          n162 = Select(t=1.0, s=w353, f=0.0) -> (s? t:f=w350:dbl)
                        }
                        n163 = script code="tube_diameters = [.01,.02,.03,.04];\naddpath('C:\\Users\\HPLC\\Dropbox (MIT)\\MoD Files\\MATLAB');\ncalculate_reactor_volumes;"("BayConfig"=w327, "Vr1"=w345, "Vr2"=w344, "Vr3"=w343, "Vr4"=w342, "Vr5"=w341, "tube_length"=w340, "tube_id"=w339, "new_len_react"=w336, "new_vol_react"=w333) -> ("Vr1"=w326:dbl, "Vr2"=w325:dbl, "Vr3"=w324:dbl, "Vr4"=w323:dbl, "Vr5"=w322:dbl)  [unwired: 1 in, 1 out]
                        n164 = local write "Vr1"(w326) -> ()
                        n165 = local write "Vr2"(w325) -> ()
                        n166 = local write "Vr3"(w324) -> ()
                        n167 = local write "Vr4"(w323) -> ()
                        n168 = local write "Vr5"(w322) -> ()
                      }
                      frame #4 {
                        n169 = local read "Setup Error"() -> (w356:bool)
                        n170 = case shown="True" w356 {
                          tunnel: [TRUE FALSE] -> w354
                          tunnel: ["" "Sytem setup has not been confirmed!"] -> w355
                          frame False {
                          }
                          frame True {
                            n171 = local read "Error Message"() -> (w361:string)
                            n172 = One Button Dialog(message=w361) -> ()  [unwired: 1 in, 1 out]
                          }
                        }
                        n173 = local write "System Confirm Not Clicked"(w355) -> ()
                        n174 = local write "Setup Confirm"(w354) -> ()
                      }
                    }
                  }
                }
              }
            }
            n175 = local read "Stop"() -> (w161:bool)
            n176 = Or(x=w162, y=w161) -> (x .or. y?=w160:bool)
            n177 = disable-structure shown="Disabled" {
              disable-tunnel: 400 -> [w168 _]
              frame Disabled {
                n178 = event shown="[1]" {
                  selector: _ -> [_ _]
                  dyn-events: _ -> [_ _]
                  timeout: w168 -> [_ _]
                  event Timeout {
                    n179 = event-data() -> ()  [unwired: 1 in, 3 out]
                  }
                  event #1 (no event record) {
                    n180 = event-data() -> ()  [unwired: 1 in, 6 out]
                    n181 = local read "Setup Confirm"() -> (w169:bool)
                    n182 = local read "Reaction Scheme Confirm"() -> (w170:bool)
                    n183 = Not(x=w169) -> (.not. x?=w172:bool)
                    n184 = And(x=w170, y=w172) -> (x .and. y?=w171:bool)
                    n185 = case shown="True" w171 {
                      frame False {
                      }
                      frame True {
                        w174 = u16 0 items=["                     Bypass", "                Hot Reactor", "                 Separator"] ("BAY 5")
                        w175 = u16 0 items=["                     Bypass", "                Hot Reactor", "                  Separator"] ("BAY 4")
                        w176 = u16 0 items=["                     Bypass", "                 Hot Reactor", "                  Separator"] ("BAY 3")
                        w177 = u16 0 items=["                     Bypass", "                Hot Reactor", "                  Separator"] ("BAY 2")
                        w178 = u16 0 items=["                 Bypass", "             Hot Reactor", "               Separator"] ("BAY 1")
                        n186 = local write "BAY 3"(w176) -> ()
                        n187 = local write "BAY 4"(w175) -> ()
                        n188 = local write "BAY 5"(w174) -> ()
                        n189 = local write "BAY 2"(w177) -> ()
                        n190 = local write "BAY 1"(w178) -> ()
                        n191 = local write "Synthesis Route Array"(string[][] [["3-Br-Pyridine _ Biphenyl", "K2CO3", "PhB(OH)2", "", "", ""]] ("Synthesis Route Array")) -> ()
                      }
                    }
                  }
                }
              }
              frame Enabled {
              }
            }
            n192 = disable-structure shown="Disabled" {
              disable-tunnel: 400 -> [w164 _]
              frame Disabled {
                n193 = event shown="[1]" {
                  selector: _ -> [_ _]
                  dyn-events: _ -> [_ _]
                  timeout: w164 -> [_ _]
                  event Timeout {
                    n194 = event-data() -> ()  [unwired: 1 in, 3 out]
                  }
                  event #1 (no event record) {
                    n195 = event-data() -> ()  [unwired: 1 in, 6 out]
                    n196 = call "File Dialog"("prompt"="Load previously saved xml file") -> ("selected path"=w166:path)  [unwired: 11 in, 3 out]
                    n197 = Path To String(path=w166) -> (string=w165:string)
                    n198 = script code="xmlDoc = xmlread(file_path);\nroot = xmlDoc.getDocumentElement();\nb = root.getChildNodes;\nrecipe = b.getElementsByTagName('Bay1').item(0);"("file_path"=w165) -> ()  [unwired: 1 in, 1 out]
                  }
                }
              }
              frame Enabled {
              }
            }
          }
        }
        frame #1 {
          n199 = local read "Stop"() -> (w363:bool)
          n200 = Not(x=w363) -> (.not. x?=w362:bool)
          n201 = case shown="True" w362 {
            tunnel: w364 -> [_ w367]
            frame False {
              "stop_button clicked" <- TRUE ("stop_button clicked")
            }
            frame True {
              # "Parameters Initilization"
              n202 = flat-sequence {
                tunnel: w367 -> [w369]
                tunnel: [w368] -> w366
                tunnel: w366 -> [w524]
                frame #0 {
                  # "Setup bays(RFID - verify)"
                  n203 = disable-structure shown="Disabled" {
                    frame Disabled {
                      n204 = local read "BAY 1"() -> ()  [unwired: 1 out]
                      n205 = local read "BAY 2"() -> ()  [unwired: 1 out]
                      n206 = local read "BAY 3"() -> ()  [unwired: 1 out]
                      n207 = local read "BAY 4"() -> ()  [unwired: 1 out]
                      n208 = local read "BAY 5"() -> ()  [unwired: 1 out]
                    }
                    frame Enabled {
                    }
                  }
                }
                frame #1 {
                  n209 = while {
                    tunnel: w369 -> [w372]
                    tunnel: [w371] -> w368
                    stop <- w375 stop-if-true
                    n210 = flat-sequence {
                      tunnel: [w385] -> w371
                      tunnel: w372 -> [w466]
                      tunnel: [w384] -> w370
                      frame #0 {
                        n211 = while {
                          stop <- w379 stop-if-true
                          n212 = event shown="[1] \"System Parameters Confirm Button\": Value Change" {
                            selector: _ -> [_ _]
                            dyn-events: _ -> [_ _]
                            timeout: u32 200 ("milliseconds to wait") -> [_ _]
                            tunnel: [FALSE TRUE] -> w377
                            event Timeout {
                              n213 = event-data() -> ()  [unwired: 1 in, 3 out]
                            }
                            event "System Parameters Confirm Button": Value Change {
                              n214 = event-data() -> ()  [unwired: 1 in, 5 out]
                              n215 = local write "System Parameters Confirm Button"(FALSE) -> ()
                            }
                          }
                          n216 = Wait (ms)(milliseconds to wait=u32 500) -> ()  [unwired: 1 out]
                          n217 = local read "Stop"() -> (w380:bool)
                          n218 = Or(x=w380, y=w377) -> (x .or. y?=w379:bool)
                        }
                      }
                      frame #1 {
                        w405 = 0 ("disabled index (col)")
                        w417 = 1 ("disabled index (col)")
                        # "Do while parameters have not been correctly entered"
                        n219 = local read "Bay Parameters"() -> (w404:T2)
                        n220 = local read "Synthesis Route Array"() -> (w418:string[][])
                        n221 = local read "Total Number of Experiments"() -> (w437:dbl)
                        n222 = Unbundle By Name(w404) -> ("Continue from previous optimization?"=w465:bool)
                        n223 = Unbundle By Name(w404) -> ("Excel File Name"=w467:string)
                        n224 = Unbundle By Name(w404) -> ("Matlab File"=w463:string)
                        n225 = Unbundle By Name(w404) -> ("Bay 1.Run at set flowrate"=w509:bool)
                        n226 = Unbundle By Name(w404) -> ("Bay 1.Pump 1 Flowrate"=w515:dbl)
                        n227 = Unbundle By Name(w404) -> ("Bay 1.Pump 2 Flowrate"=w514:dbl)
                        n228 = Unbundle By Name(w404) -> ("Bay 2.Run at set flowrate"=w507:bool)
                        n229 = Unbundle By Name(w404) -> ("Bay 2.Pump 3 Flowrate"=w513:dbl)
                        n230 = Unbundle By Name(w404) -> ("Bay 3.Pump 4 Flowrate"=w512:dbl)
                        n231 = Unbundle By Name(w404) -> ("Bay 3.Run at set flowrate"=w506:bool)
                        n232 = Unbundle By Name(w404) -> ("Bay 4.Run at set flowrate"=w503:bool)
                        n233 = Unbundle By Name(w404) -> ("Bay 4.Pump 5 Flowrate"=w511:dbl)
                        n234 = Unbundle By Name(w404) -> ("Bay 5.Pump 6 Flowrate"=w510:dbl)
                        n235 = Unbundle By Name(w404) -> ("Bay 5.Run at set flowrate"=w502:bool)
                        n236 = Index Array(array=w418, index (row)=3, index (col)=w417) -> (element=w411:string)
                        n237 = Index Array(array=w418, index (row)=2, index (col)=w417) -> (element=w409:string)
                        n238 = Index Array(array=w418, index (row)=1, index (col)=w417) -> (element=w407:string)
                        n239 = Index Array(array=w418, index (row)=0, index (col)=w417) -> (element=w420:string)
                        n240 = Index Array(array=w418, index (row)=4, index (col)=w417) -> (element=w413:string)
                        n241 = Index Array(array=w418, index (row)=5, index (col)=w417) -> (element=w415:string)
                        n242 = Build Array(w420, w407, w409, w411, w413, w415) -> (w421:string[])
                        n243 = Index Array(array=w418, index (row)=0 ("index"), index (col)=w405) -> (element=w443:string)
                        n244 = for {
                          tunnel: w421 -> [w517] mode=indexing
                          tunnel: [w516] -> w406 mode=indexing
                          n245 = script code="ctemp1 = str2num(c_temp);"("c_temp"=w517) -> ("ctemp1"=w516:dbl)  [unwired: 1 in, 1 out]
                        }
                        n246 = Boolean To (0,1)(Boolean=w507) -> (0, 1=w462:i16)
                        n247 = Boolean To (0,1)(Boolean=w503) -> (0, 1=w504:i16)
                        n248 = Boolean To (0,1)(Boolean=w506) -> (0, 1=w505:i16)
                        n249 = Boolean To (0,1)(Boolean=w465) -> (0, 1=w464:i16)
                        n250 = Boolean To (0,1)(Boolean=w509) -> (0, 1=w508:i16)
                        n251 = Boolean To (0,1)(Boolean=w502) -> (0, 1=w501:i16)
                        n252 = Index Array(array=w418, index (row)=1 ("index"), index (col)=w405) -> (element=w438:string)
                        n253 = Index Array(array=w418, index (row)=2 ("index"), index (col)=w405) -> (element=w439:string)
                        n254 = Unbundle By Name(w404) -> ("Bay 1.optimize_temp"=w500:bool)
                        n255 = Unbundle By Name(w404) -> ("Bay 1.optimize_tau"=w498:bool)
                        n256 = Unbundle By Name(w404) -> ("Bay 2.optimize_temp"=w496:bool)
                        n257 = Unbundle By Name(w404) -> ("Bay 2.optimize_tau"=w494:bool)
                        n258 = Unbundle By Name(w404) -> ("Bay 3.optimize_temp"=w492:bool)
                        n259 = Unbundle By Name(w404) -> ("Bay 3.optimize_tau"=w490:bool)
                        n260 = Unbundle By Name(w404) -> ("Bay 4.optimize_temp"=w488:bool)
                        n261 = Unbundle By Name(w404) -> ("Bay 4.optimize_tau"=w486:bool)
                        n262 = Index Array(array=w418, index (row)=3 ("index"), index (col)=w405) -> (element=w440:string)
                        n263 = Boolean To (0,1)(Boolean=w488) -> (0, 1=w487:i16)
                        n264 = Boolean To (0,1)(Boolean=w486) -> (0, 1=w485:i16)
                        n265 = Index Array(array=w418, index (row)=4 ("index"), index (col)=w405) -> (element=w441:string)
                        n266 = Boolean To (0,1)(Boolean=w490) -> (0, 1=w489:i16)
                        n267 = Boolean To (0,1)(Boolean=w496) -> (0, 1=w495:i16)
                        n268 = Boolean To (0,1)(Boolean=w500) -> (0, 1=w499:i16)
                        n269 = Boolean To (0,1)(Boolean=w494) -> (0, 1=w493:i16)
                        n270 = Boolean To (0,1)(Boolean=w498) -> (0, 1=w497:i16)
                        n271 = Boolean To (0,1)(Boolean=w492) -> (0, 1=w491:i16)
                        n272 = Unbundle By Name(w404) -> ("Bay 5.optimize_temp"=w484:bool)
                        n273 = Unbundle By Name(w404) -> ("Bay 5.optimize_tau"=w482:bool)
                        n274 = Index Array(array=w418, index (row)=5 ("index"), index (col)=w405) -> (element=w442:string)
                        n275 = Boolean To (0,1)(Boolean=w484) -> (0, 1=w483:i16)
                        n276 = Boolean To (0,1)(Boolean=w482) -> (0, 1=w481:i16)
                        n277 = Build Array(w499, w497, w495, w493, w491, w489, w487, w485, w483, w481) -> (w480:i16[])
                        n278 = Unbundle By Name(w404) -> ("Bay 1.Temperature Params"=w477:dbl[])
                        n279 = Unbundle By Name(w404) -> ("Bay 2.Temperature Params"=w476:dbl[])
                        n280 = Unbundle By Name(w404) -> ("Bay 2.Resisdence time params"=w471:dbl[])
                        n281 = Unbundle By Name(w404) -> ("Bay 3.Temperature Params"=w475:dbl[])
                        n282 = Unbundle By Name(w404) -> ("Bay 3.Resisdence time params"=w470:dbl[])
                        n283 = Unbundle By Name(w404) -> ("Bay 4.Temperature Params"=w474:dbl[])
                        n284 = Unbundle By Name(w404) -> ("Bay 4.Resisdence time params"=w469:dbl[])
                        n285 = Unbundle By Name(w404) -> ("Bay 5.Temperature Params"=w473:dbl[])
                        n286 = Unbundle By Name(w404) -> ("Bay 5.Resisdence time params"=w468:dbl[])
                        n287 = Unbundle By Name(w404) -> ("Bay 1.pump params 2"=w436:dbl[])
                        n288 = Unbundle By Name(w404) -> ("Bay 1.pump params 1"=w472:dbl[])
                        n289 = Unbundle By Name(w404) -> ("Bay 1.Run at set temperature"=w427:bool)
                        n290 = Unbundle By Name(w404) -> ("Bay 2.Run at set temperature"=w425:bool)
                        n291 = Unbundle By Name(w404) -> ("Bay 3.Run at set temperature"=w424:bool)
                        n292 = Unbundle By Name(w404) -> ("Bay 4.Run at set temperature"=w423:bool)
                        n293 = Unbundle By Name(w404) -> ("Bay 5.Run at set temperature"=w422:bool)
                        n294 = Unbundle By Name(w404) -> ("Bay 3.Temperature"=w433:dbl)
                        n295 = Unbundle By Name(w404) -> ("Bay 1.Temperature"=w435:dbl)
                        n296 = Unbundle By Name(w404) -> ("Bay 2.Temperature"=w434:dbl)
                        n297 = Unbundle By Name(w404) -> ("Bay 4.Temperature"=w432:dbl)
                        n298 = Unbundle By Name(w404) -> ("Bay 5.Temperature"=w431:dbl)
                        n299 = Unbundle By Name(w404) -> ("Bay 3.pump_num_ratio"=w456:dbl)
                        n300 = Unbundle By Name(w404) -> ("Bay 4.pump_num_ratio"=w453:dbl)
                        n301 = Unbundle By Name(w404) -> ("Bay 5.pump_num_ratio"=w450:dbl)
                        n302 = Unbundle By Name(w404) -> ("Bay 2.pump_num_ratio"=w459:dbl)
                        n303 = Unbundle By Name(w404) -> ("Bay 4.pump_at_ratio"=w455:bool)
                        n304 = Boolean To (0,1)(Boolean=w455) -> (0, 1=w454:i16)
                        n305 = Unbundle By Name(w404) -> ("Bay 3.pump_at_ratio"=w458:bool)
                        n306 = Boolean To (0,1)(Boolean=w458) -> (0, 1=w457:i16)
                        n307 = Unbundle By Name(w404) -> ("Bay 5.pump_at_ratio"=w452:bool)
                        n308 = Boolean To (0,1)(Boolean=w452) -> (0, 1=w451:i16)
                        n309 = Unbundle By Name(w404) -> ("Bay 2.pump_at_ratio"=w461:bool)
                        n310 = Boolean To (0,1)(Boolean=w461) -> (0, 1=w460:i16)
                        n311 = Build Array(w435, w434, w433, w432, w431) -> (w430:dbl[])
                        n312 = Build Array(w427, w425, w424, w423, w422) -> (w426:bool[])
                        n313 = for {
                          N: 5 -> [_]
                          tunnel: w426 -> [w521] mode=indexing
                          tunnel: [w520] -> w428 mode=indexing
                          n314 = Select(t=1.0, s=w521, f=0.0) -> (s? t:f=w520:dbl)
                        }
                        n315 = Unbundle By Name(w404) -> ("Internal Standard?"=w395:bool)
                        n316 = Unbundle By Name(w404) -> ("increas_decrease_hplc_peak"=w396:bool)
                        n317 = Unbundle By Name(w404) -> ("Hplc Wait time(min)"=w388:dbl)
                        n318 = Unbundle By Name(w404) -> ("Total Number of Experiments 2"=w387:dbl)
                        n319 = Unbundle By Name(w404) -> ("hplc_start"=w392:dbl)
                        n320 = Unbundle By Name(w404) -> ("ISTD start"=w390:dbl)
                        n321 = Unbundle By Name(w404) -> ("hplc_end"=w391:dbl)
                        n322 = Unbundle By Name(w404) -> ("throughput_yield"=w397:bool)
                        n323 = Unbundle By Name(w404) -> ("ISTD end"=w389:dbl)
                        n324 = Select(t=1.0, s=w396, f=0.0) -> (s? t:f=w394:dbl)
                        n325 = Select(t=1.0, s=w395, f=0.0) -> (s? t:f=w393:dbl)
                        n326 = Select(t=0.0, s=w397, f=1.0) -> (s? t:f=w386:dbl)
                        n327 = script code="system_error = 0;\nnumPeaks = 1;\nstart_phase_time = 1;\nis_redo_exp = 0;\nFvalues = [];\nHPLC_Area = [];\n\nT1_span = [1 1]; T2_span = [1 1]; T3_span = [1 1]; T4_span = [1 1]; T5_span = [1 1];\nT_span = [T1_span;T2_span;T3_span;T4_span;T5_span];\n p1_span =  [1 1]; p2_span =  [1 1]; p3_span =  [1 1]; p4_span =  [1 1]; p5_span =  [1 1];  p6_span =  [1 1];\nOpt_params = [0 0 0 0 0 0 0 0 0 0 0];\nT_params = [T1_params;T2_params;T3_params;T4_params;T5_params];\npump_params = [pump1_params;pump2_params;pump3_params;pump4_params;pump5_params;pump6_params];\nopt_ctr = 0;ncall = 100;record_data = true;\nT1_SP = 23; T2_SP = 23; T3_SP = 23; T4_SP = 23; T5_SP = 23;\nT_span = [T1_span;T2_span;T3_span;T4_span;T5_span];\np_span = [p1_span;p2_span;p3_span;p4_span;p5_span;p6_span];\nno_errors = 1;\nP1 = 0; P2 =0; P3 = 0; P4 = 0; P5 = 0; P6 = 0;\nP = [P1, P2, P3,P4, P5, P6];\nis_first_set_of_exp = true;\nerror_message = 'System has no errors to report';\naddpath(genpath('C:\\Users\\HPLC\\Dropbox (MIT)\\MoD Files\\MATLAB'))\naddpath(genpath('C:\\Users\\Admin\\Dropbox (MIT)\\MoD Files\\MATLAB'))\nallMSData = [];allHPLCData = [];allHPLCFile = [];\nBay_ratio = [0,Bay2_ratio,Bay3_ratio,Bay4_ratio,Bay5_ratio];\nBay_pump_ratio = [1, Bay2_pump_ratio, Bay3_pump_ratio, Bay4_pump_ratio, Bay5_pump_ratio];\nP_setrate = [P1_setrate, P2_setrate, P3_setrate, P4_setrate, P5_setrate, P6_setrate];\nuse_flowrate = [use_flowrate1, use_flowrate2,use_flowrate3, use_flowrate4, use_flowrate5];\npump_chem_name= []\nCurrExp = 1;\n% ****************************************************************************************************\n%Setup optimization\n   setup_optimization_params;\n   initialize_opt = 0;\n   nstop0 = 0;\n%*****************************************************************************************************\n% Setup excel and xml file writing\npath(path, pa);\nnumMSSig = 1;\nsetup_excel_output;\n%***************************************************************************************************\nredo = false;\nncall = ncall_in;"("use_flowrate1"=w508, "P1_setrate"=w515, "P2_setrate"=w514, "P3_setrate"=w513, "P4_setrate"=w512, "P5_setrate"=w511, "P6_setrate"=w510, "use_flowrate2"=w462, "use_flowrate3"=w505, "use_flowrate4"=w504, "use_flowrate5"=w501, "Optimize_params"=w480, "T1_params"=w477, "T2_params"=w476, "T3_params"=w475, "T4_params"=w474, "T5_params"=w473, "pump1_params"=w472, "pump3_params"=w471, "pump4_params"=w470, "pump5_params"=w469, "pump6_params"=w468, "xl_file"=w467, "pa"=w466, "Continue"=w464, "matlabsavefile"=w463, "Bay2_ratio"=w460, "Bay2_pump_ratio"=w459, "Bay3_ratio"=w457, "Bay3_pump_ratio"=w456, "Bay4_ratio"=w454, "Bay4_pump_ratio"=w453, "Bay5_ratio"=w451, "Bay5_pump_ratio"=w450, "pump1_chem"=w443, "pump6_chem"=w442, "pump5_chem"=w441, "pump4_chem"=w440, "pump3_chem"=w439, "pump2_chem"=w438, "Pump_concen"=w406, "ncall_in"=w437, "pump2_params"=w436, "T_SP"=w430, "Run_at_T_SP"=w428, "incr_hplc_peak"=w394, "use_internal_std"=w393, "hplc_peak_start"=w392, "hplc_peak_end"=w391, "ISTD_start"=w390, "ISTD_end"=w389, "hplc_wait_time"=w388, "tot_num_exp"=w387, "throughput_yield"=w386) -> ("no_errors"=w479:dbl, "error_message"=w478:string)  [unwired: 1 in, 1 out]
                        n328 = Not Equal To 0?(x=w479) -> (x != 0?=w384:bool)
                        n329 = Not(x=w384) -> (.not. x?=w385:bool)
                        n330 = case shown="False" w385 {
                          tunnel: w478 -> [_ w523]
                          frame False {
                            n331 = local write "Setup Confirm 2"(TRUE ("Setup Confirm 2")) -> ()
                          }
                          frame True {
                            n332 = One Button Dialog(message=w523) -> ()  [unwired: 1 in, 1 out]
                          }
                        }
                      }
                    }
                    n333 = local read "Stop"() -> (w374:bool)
                    n334 = Or(x=w370, y=w374) -> (x .or. y?=w375:bool)
                    n335 = Wait (ms)(milliseconds to wait=u32 500) -> ()  [unwired: 1 out]
                  }
                }
                frame #2 {
                  n336 = local write "System Error"(w524) -> ()
                }
              }
            }
          }
        }
        frame #2 {
          # "Run Initial diagnostics"
        }
        frame #3 {
          # "Run System"
          n337 = while {
            stop <- w1135 stop-if-true
            n338 = local read "Debug_run_button"() -> (w1131:bool)
            n339 = Not(x=w1131) -> (.not. x?=w1133:bool)
            n340 = local read "Temperature Control 1"() -> (w1130:bool)
            n341 = And(x=w1133, y=w1130) -> (x .and. y?=w1132:bool)
            n342 = case shown="True" w1132 {
              frame False {
                n343 = local write "Temp SS? 1"(TRUE ("Temp SS? 1")) -> ()
              }
              frame True {
                # "Bay 1 Temperature Controller"
                n344 = local read "Temperature SP 1"() -> (w1137:dbl)
                n345 = local read "Temperature 1"() -> (w1141:dbl)
                n346 = local read "SSR Duration 1"() -> (w1156:dbl)
                n347 = call-poly <vilib>:"PID Online Autotuning.vi"("setpoint"=w1137, "manipulated variable"=w1156, "autotuning parameters"=T9 {"type of controller"=enum."PID", "relay cycles"=3, "relay amplitude"=1.0, "control specifications"=enum."Normal", "PV noise level"=0.1} ("Autotuning Parameters R1"), "process variable"=w1141, "PID gains in"=T8 {"Proportional gain Kc"=0.38538, "Integral time Ti (sec)"=0.524375, "Derivative time Ti (sec)"=0.12585} ("PID gains 2")) -> ("setpoint out"=w1162:dbl, "process variable out"=w1161:dbl, "PID gains out"=w1158:T11)  [unwired: 6 in, 2 out]
                n348 = call <vilib>:"PID Autotuning (Temperature).vi"("desired temperature"=w1162, "measured temperature"=w1161, "plant parameters in"=w1158, "output range"=cluster{"output high":dbl, "output low":dbl} {"output high"=3.0, "output low"=-1.0} ("Output range")) -> ("output"=w1154:dbl)  [unwired: 12 in, 3 out]
                n349 = local write "SSR Duration 1"(w1154) -> ()
                n350 = Subtract(x=w1137, y=w1141) -> (x-y=w1148:dbl)
                n351 = Absolute Value(x=w1148) -> (abs(x)=w1151:dbl)
                n352 = Multiply(x=1000.0, y=w1154) -> (x*y=w1152:dbl)
                n353 = Greater Than 0?(x=w1152) -> (x > 0?=w1146:bool)
                n354 = Less Or Equal?(x=w1151, y=1.2) -> (x <= y?=w1149:bool)
                n355 = Greater?(x=w1137, y=w1141) -> (0:w1147:bool)
                n356 = And(x=w1146, y=w1147) -> (x .and. y?=w1144:bool)
                n357 = local write "Temp SS? 1"(w1149) -> ()
                n358 = Subtract(x=w1141, y=10.0) -> (x-y=w1142:dbl)
                n359 = Less?(x=w1142, y=w1137) -> (x < y?=w1145:bool)
                n360 = And(x=w1145, y=w1144) -> (x .and. y?=w1143:bool)
                n361 = case shown="False" w1143 {
                  tunnel: [errorcluster {"status"=FALSE, "code"=0, "source"=""} ("error out") errorcluster {"status"=FALSE, "code"=0, "source"=""} ("error out")] -> _
                  tunnel: 2 -> [_ _]
                  tunnel: w1152 -> [w1166 _]
                  tunnel: [0.0 w1171] -> w1139
                  tunnel: w1137 -> [_ w1170]
                  frame False {
                    n362 = Absolute Value(x=w1166) -> (abs(x)=w1167:dbl)
                    n363 = Wait (ms)(milliseconds to wait=w1167) -> ()  [unwired: 1 out]
                  }
                  frame True {
                    n364 = script code="tempdiff1= SP1 - T1;\nif tempdiff1 > 10\n  if slope1 < .01\n     temp_check1 = temp_check1 + 1;\n  else\n      temp_check1 =0;\n  end\nend\n\nif temp_check1 > 9\n  temp_error1 = 1\nend"("SP1"=w1170) -> ("temp_error1"=w1171:dbl)  [unwired: 1 in, 1 out]
                  }
                }
                n365 = Not Equal To 0?(x=w1139) -> (x != 0?=w1138:bool)
                n366 = case shown="True" w1138 {
                  frame False {
                  }
                  frame True {
                    n367 = local write "Error Message"("Bay 1 Temperature Heating Error") -> ()
                  }
                }
                n368 = case shown="True" w1138 {
                  tunnel: w1138 -> [_ w1164]
                  frame False {
                  }
                  frame True {
                    n369 = local write "System Error"(w1164) -> ()
                    n370 = local write "Stop"(w1164) -> ()
                  }
                }
              }
            }
            n371 = Wait (ms)(milliseconds to wait=u32 400) -> ()  [unwired: 1 out]
            n372 = local read "Stop"() -> (w1135:bool)
          }
          n373 = local read "Bay Parameters"() -> (w528:T2)
          n374 = while {
            stop <- w1093 stop-if-true
            n375 = local read "Debug_run_button"() -> (w1089:bool)
            n376 = Not(x=w1089) -> (.not. x?=w1091:bool)
            n377 = local read "Temperature Control 2"() -> (w1088:bool)
            n378 = And(x=w1091, y=w1088) -> (x .and. y?=w1090:bool)
            n379 = case shown="True" w1090 {
              frame False {
                n380 = local write "Temp SS? 2"(TRUE ("Temp SS? 2")) -> ()
              }
              frame True {
                # "Bay 2 Temperature Controller"
                n381 = local read "Temperature SP 2"() -> (w1096:dbl)
                n382 = local read "Temperature 2"() -> (w1099:dbl)
                n383 = local read "SSR Duration 2"() -> (w1117:dbl)
                n384 = call-poly <vilib>:"PID Online Autotuning.vi"("setpoint"=w1096, "manipulated variable"=w1117, "autotuning parameters"=T9 {"type of controller"=enum."PID", "relay cycles"=3, "relay amplitude"=1.0, "control specifications"=enum."Normal", "PV noise level"=0.1} ("Autotuning Parameters R1"), "process variable"=w1099, "PID gains in"=T8 {"Proportional gain Kc"=0.38538, "Integral time Ti (sec)"=0.524375, "Derivative time Ti (sec)"=0.12585} ("PID gains 2")) -> ("setpoint out"=w1115:dbl, "process variable out"=w1114:dbl, "PID gains out"=w1120:T11)  [unwired: 6 in, 2 out]
                n385 = call <vilib>:"PID Autotuning (Temperature).vi"("desired temperature"=w1115, "measured temperature"=w1114, "plant parameters in"=w1120, "output range"=cluster{"output high":dbl, "output low":dbl} {"output high"=3.0, "output low"=-1.0} ("Output range")) -> ("output"=w1110:dbl)  [unwired: 12 in, 3 out]
                n386 = local write "SSR Duration 2"(w1110) -> ()
                n387 = Greater?(x=w1096, y=w1099) -> (0:w1105:bool)
                n388 = Multiply(x=1000.0, y=w1110) -> (x*y=w1112:dbl)
                n389 = Greater Than 0?(x=w1112) -> (x > 0?=w1104:bool)
                n390 = And(x=w1104, y=w1105) -> (x .and. y?=w1102:bool)
                n391 = Subtract(x=w1096, y=w1099) -> (x-y=w1107:dbl)
                n392 = Absolute Value(x=w1107) -> (abs(x)=w1109:dbl)
                n393 = Subtract(x=w1099, y=10.0) -> (x-y=w1101:dbl)
                n394 = Less Or Equal?(x=w1109, y=1.2) -> (x <= y?=w1106:bool)
                n395 = local write "Temp SS? 2"(w1106) -> ()
                n396 = Less?(x=w1101, y=w1096) -> (x < y?=w1103:bool)
                n397 = And(x=w1103, y=w1102) -> (x .and. y?=w1098:bool)
                n398 = case shown="False" w1098 {
                  tunnel: [errorcluster {"status"=FALSE, "code"=0, "source"=""} ("error out") errorcluster {"status"=FALSE, "code"=0, "source"=""} ("error out")] -> _
                  tunnel: 3 -> [_ _]
                  tunnel: w1112 -> [w1124 _]
                  tunnel: [0.0 w1129] -> w1097
                  tunnel: w1096 -> [_ w1128]
                  frame False {
                    n399 = Absolute Value(x=w1124) -> (abs(x)=w1125:dbl)
                    n400 = Wait (ms)(milliseconds to wait=w1125) -> ()  [unwired: 1 out]
                  }
                  frame True {
                    n401 = script code="tempdiff2= SP2 - T2;\nif tempdiff2 > 10\n  if slope2 < .01\n     temp_check2 = temp_check2 + 1;\n  else\n      temp_check2 =0;\n  end\nend\n\nif temp_check2 > 9\n  temp_error2 = 1\nend"("SP2"=w1128) -> ("temp_error2"=w1129:dbl)  [unwired: 1 in, 1 out]
                  }
                }
                n402 = Not Equal To 0?(x=w1097) -> (x != 0?=w1095:bool)
                n403 = case shown="True" w1095 {
                  frame False {
                  }
                  frame True {
                    n404 = local write "Error Message"("Bay 2 Temperature Heating Error") -> ()
                  }
                }
                n405 = case shown="True" w1095 {
                  tunnel: w1095 -> [_ w1122]
                  frame False {
                  }
                  frame True {
                    n406 = local write "Stop"(w1122) -> ()
                    n407 = local write "System Error"(w1122) -> ()
                  }
                }
              }
            }
            n408 = local read "Stop"() -> (w1093:bool)
            n409 = Wait (ms)(milliseconds to wait=u32 400) -> ()  [unwired: 1 out]
          }
          n410 = local read "Stop"() -> (w525:bool)
          n411 = Not(x=w525) -> (.not. x?=w527:bool)
          n412 = case shown="True" w527 {
            tunnel: w528 -> [_ w532]
            tunnel: w526 -> [_ w531]
            frame False {
            }
            frame True {
              n413 = while {
                tunnel: w532 -> [w545]
                tunnel: w531 -> [w537]
                i -> [w544]
                stop <- w538 stop-if-true
                n414 = local read "running?"() -> (w533:bool)
                n415 = Wait (ms)(milliseconds to wait=u32 1000) -> ()  [unwired: 1 out]
                n416 = Increment(x=w544) -> (x+1=w534:i32)
                n417 = case shown="True" w533 {
                  tunnel: w544 -> [w550 _]
                  tunnel: w545 -> [_ _]
                  tunnel: [w552 w555] -> w535
                  tunnel: [0.0 w556] -> w540
                  tunnel: w537 -> [_ w554]
                  frame False {
                    # "STANDBY MODE"
                    n418 = Add(x=w550, y=2.0) -> (x+y=w552:dbl)
                  }
                  frame True {
                    n419 = flat-sequence {
                      tunnel: w554 -> [w558]
                      tunnel: [w558] -> w553
                      tunnel: [w566] -> w556
                      tunnel: [200.0] -> w555
                      tunnel: w553 -> [w564]
                      frame #0 {
                        n420 = local write "stop_xl_write"(FALSE ("stop_xl_write")) -> ()
                      }
                      frame #1 {
                        # "Increase flowrate of dilution stream"
                        # "Wait mixed stream reaches SL"
                        # "SNOBFIT"
                        # "Optimize"
                        # "Run Experimental Conditions"
                        # "Optimize/Synthesize"
                        n421 = local read "Stop"() -> (w561:bool)
                        n422 = Not(x=w561) -> (.not. x?=w560:bool)
                        n423 = case shown="True" w560 {
                          tunnel: [1.0 w583] -> w569
                          tunnel: [w577 w582] -> w563
                          tunnel: [0.0 w581] -> w562
                          tunnel: [w577 w580] -> w559
                          frame False {
                            w577 = dbl[] []
                          }
                          frame True {
                            n424 = script code="optimization_main_loop"() -> ("Conditions_Array"=w582:dbl[], "opt_ctr"=w583:dbl, "P_tot"=w581:dbl, "tau_array"=w580:dbl[])  [unwired: 1 in, 1 out]
                          }
                        }
                        "P_tot" <- w562
                        n425 = local read "COMM Port :: Milligat Pumps"() -> (w570:refnum<visa-resource-name>)
                        n426 = Equal?(x=w569, y=1.0) -> (x = y?=w567:bool)
                        n427 = flat-sequence {
                          tunnel: w563 -> [w945]
                          tunnel: w559 -> [w939]
                          frame #0 {
                            # "Start recording data"
                            n428 = Index Array(array=w945, index=5) -> (element=w957:dbl)
                            n429 = Index Array(array=w945, index=0) -> (element=w952:dbl)
                            n430 = Index Array(array=w945, index=1) -> (element=w953:dbl)
                            n431 = Index Array(array=w945, index=2) -> (element=w955:dbl)
                            n432 = Index Array(array=w945, index=3) -> (element=w954:dbl)
                            n433 = Index Array(array=w945, index=4) -> (element=w956:dbl)
                            n434 = local write "Pump setpoint(ul/min) 2"(w953) -> ()
                            n435 = local write "Pump setpoint(ul/min) 4"(w955) -> ()
                            n436 = local write "Pump setpoint(ul/min) 5"(w956) -> ()
                            n437 = local write "Pump setpoint(ul/min) 3"(w954) -> ()
                            n438 = local write "Pump setpoint(ul/min) 6"(w957) -> ()
                            n439 = local write "Pump setpoint(ul/min) 1"(w952) -> ()
                            n440 = Index Array(array=w939, index=0) -> (element=w944:dbl)
                            n441 = Index Array(array=w939, index=4) -> (element=w943:dbl)
                            n442 = Index Array(array=w939, index=3) -> (element=w942:dbl)
                            n443 = Index Array(array=w939, index=2) -> (element=w941:dbl)
                            n444 = Index Array(array=w939, index=1) -> (element=w940:dbl)
                            n445 = local write "tau 2"(w940) -> ()
                            n446 = local write "tau 3"(w941) -> ()
                            n447 = local write "tau 4"(w942) -> ()
                            n448 = local write "tau 5"(w943) -> ()
                            n449 = local write "tau 1"(w944) -> ()
                          }
                        }
                        n450 = flat-sequence {
                          tunnel: w570 -> [w587]
                          tunnel: w563 -> [w586]
                          tunnel: w567 -> [w585]
                          tunnel: [w585] -> w576
                          tunnel: w564 -> [w584]
                          tunnel: w576 -> [w696]
                          tunnel: [w696] -> w575
                          tunnel: w575 -> [w716]
                          tunnel: [w714] -> w574
                          tunnel: w563 -> [w737]
                          tunnel: w574 -> [w736]
                          tunnel: [w878] -> w573
                          tunnel: w573 -> [w891]
                          tunnel: [w891] -> w572
                          tunnel: w572 -> [w899]
                          tunnel: [w899] -> w571
                          tunnel: [w933] -> w566
                          tunnel: w571 -> [w933]
                          frame #0 {
                            # "Setup pump flowrates and temperature setpoints"
                            n451 = stacked-sequence {
                              tunnel: w587 -> [w609 _ _ _ _]
                              tunnel: w587 -> [_ w634 _ _ _]
                              tunnel: w587 -> [_ _ w653 _ _]
                              tunnel: w587 -> [_ _ _ w672 _]
                              tunnel: w587 -> [_ _ _ _ w691]
                              tunnel: w586 -> [w606 w632 w651 w670 w688]
                              tunnel: w585 -> [w596 w625 w644 w663 w682]
                              tunnel: w584 -> [w594 _ _ _ _]
                              frame #0 {
                                # "Bay 1"
                                n452 = local read "Syringe_pump?"() -> (w595:bool)
                                n453 = Index Array(array=w606, index=0) -> (element=w604:dbl)
                                n454 = local read "BAY 1"() -> (w589:u16)
                                n455 = Index Array(array=w606, index=1) -> (element=w603:dbl)
                                n456 = Index Array(array=w606, index=6) -> (element=w602:dbl)
                                n457 = script code="MATLAB script"("P1"=w604, "P2"=w603, "T1_SP"=w602) -> ()  [unwired: 1 in, 1 out]
                                n458 = Less Or Equal?(x=w589, y=u16 4) -> (x <= y?=w591:bool)
                                n459 = Greater Or Equal?(x=w589, y=u16 1) -> (x >= y?=w592:bool)
                                n460 = And(x=w592, y=w591) -> (x .and. y?=w593:bool)
                                n461 = Greater Than 0?(x=w604) -> (x > 0?=w601:bool)
                                n462 = And(x=w601, y=w596) -> (x .and. y?=w600:bool)
                                n463 = Greater Than 0?(x=w603) -> (x > 0?=w599:bool)
                                n464 = And(x=w599, y=w596) -> (x .and. y?=w598:bool)
                                n465 = And(x=w593, y=w596) -> (x .and. y?=w597:bool)
                                n466 = case shown="True" w595 {
                                tunnel: w609 -> [w612 _]
                                tunnel: w603 -> [w611 w614]
                                tunnel: w598 -> [w610 w615]
                                tunnel: w594 -> [_ w613]
                                frame False {
                                n467 = case shown="False" w610 {
                                tunnel: w612 -> [_ _]
                                tunnel: w611 -> [_ _]
                                frame False {
                                }
                                frame True {
                                }
                                }
                                }
                                frame True {
                                n468 = case shown="True" w615 {
                                tunnel: w614 -> [_ _]
                                tunnel: w613 -> [_ _]
                                frame False {
                                }
                                frame True {
                                (unwired) u16 0 items=["Infuse", "Withdraw"] ("Run Direction (0:Infuse)")
                                (unwired) u32 4 items=["milliliters per hour (ml/hr)", "milliliters per minute (ml/min)", "milliliters per second (ml/sec)", "microliters per hour (ul/hr)", "microliters per minute (ul/min)", "microliters per second (ul/sec)", "nanoliters per hour (nl/hr)", "nanoliters per minute (nl/min)", "nanoliters per second (nl/sec)", "picoliters per hour (pl/hr)", "picoliters per minute (pl/min)", "picoliters per second (pl/sec)"] ("Flow Rate Units (1:ml/min)")
                                (unwired) u16 0 items=["Infuse", "Withdraw"] ("Pump Direction (0:Infuse)")
                                }
                                }
                                }
                                }
                                n469 = case shown="False" w600 {
                                tunnel: w609 -> [_ _]
                                tunnel: w604 -> [_ _]
                                frame False {
                                }
                                frame True {
                                # "switched j and g"
                                }
                                }
                                n470 = case shown="True" w597 {
                                tunnel: w602 -> [_ w618]
                                frame False {
                                n471 = local write "Temperature Control 1"(FALSE) -> ()
                                }
                                frame True {
                                n472 = local write "Temperature SP 1"(w618) -> ()
                                n473 = local write "Temperature Control 1"(TRUE ("Temperature Control 1")) -> ()
                                }
                                }
                              }
                              frame #1 {
                                # "Bay 2"
                                n474 = local read "BAY 2"() -> (w621:u16)
                                n475 = Index Array(array=w632, index=2) -> (element=w629:dbl)
                                n476 = Index Array(array=w632, index=7) -> (element=w630:dbl)
                                n477 = script code="MATLAB script"("T2_SP"=w630, "P3"=w629) -> ()  [unwired: 1 in, 1 out]
                                n478 = Greater Than 0?(x=w629) -> (x > 0?=w627:bool)
                                n479 = And(x=w627, y=w625) -> (x .and. y?=w626:bool)
                                n480 = Greater Or Equal?(x=w621, y=u16 1) -> (x >= y?=w619:bool)
                                n481 = Less Or Equal?(x=w621, y=u16 4) -> (x <= y?=w624:bool)
                                n482 = And(x=w619, y=w624) -> (x .and. y?=w623:bool)
                                n483 = And(x=w623, y=w625) -> (x .and. y?=w628:bool)
                                n484 = case shown="True" w628 {
                                tunnel: w630 -> [_ w636]
                                frame False {
                                n485 = local write "Temperature Control 2"(FALSE) -> ()
                                }
                                frame True {
                                n486 = local write "Temperature Control 2"(TRUE ("Temperature Control 2")) -> ()
                                n487 = local write "Temperature SP 2"(w636) -> ()
                                }
                                }
                                n488 = case shown="True" w626 {
                                tunnel: w629 -> [_ _]
                                tunnel: w634 -> [_ _]
                                frame False {
                                }
                                frame True {
                                }
                                }
                              }
                              frame #2 {
                                # "Bay 3"
                                n489 = local read "BAY 3"() -> (w639:u16)
                                n490 = Index Array(array=w651, index=3) -> (element=w648:dbl)
                                n491 = Not Equal To 0?(x=w648) -> (x != 0?=w647:bool)
                                n492 = Index Array(array=w651, index=8) -> (element=w649:dbl)
                                n493 = script code="MATLAB script"("T3_SP"=w649, "P4"=w648) -> ()  [unwired: 1 in, 1 out]
                                n494 = Less Or Equal?(x=w639, y=u16 4) -> (x <= y?=w643:bool)
                                n495 = Greater Or Equal?(x=w639, y=u16 1) -> (x >= y?=w640:bool)
                                n496 = And(x=w640, y=w643) -> (x .and. y?=w638:bool)
                                n497 = And(x=w638, y=w644) -> (x .and. y?=w645:bool)
                                n498 = And(x=w647, y=w644) -> (x .and. y?=w646:bool)
                                n499 = case shown="True" w646 {
                                tunnel: w648 -> [_ _]
                                tunnel: w653 -> [_ _]
                                frame False {
                                }
                                frame True {
                                }
                                }
                                n500 = case shown="False" w645 {
                                tunnel: w649 -> [_ w655]
                                frame False {
                                n501 = local write "Temperature Control 3"(FALSE) -> ()
                                }
                                frame True {
                                n502 = local write "Temperature Control 3"(TRUE ("Temperature Control 3")) -> ()
                                n503 = local write "Temperature SP 3"(w655) -> ()
                                }
                                }
                              }
                              frame #3 {
                                # "Bay 4"
                                n504 = Index Array(array=w670, index=9) -> (element=w667:dbl)
                                n505 = Index Array(array=w670, index=4) -> (element=w668:dbl)
                                n506 = script code="MATLAB script"("P5"=w668, "T4_SP"=w667) -> ()  [unwired: 1 in, 1 out]
                                n507 = Not Equal To 0?(x=w668) -> (x != 0?=w666:bool)
                                n508 = local read "BAY 4"() -> (w657:u16)
                                n509 = And(x=w666, y=w663) -> (x .and. y?=w665:bool)
                                n510 = Less Or Equal?(x=w657, y=u16 4) -> (x <= y?=w662:bool)
                                n511 = Greater Or Equal?(x=w657, y=u16 1) -> (x >= y?=w659:bool)
                                n512 = And(x=w659, y=w662) -> (x .and. y?=w658:bool)
                                n513 = And(x=w658, y=w663) -> (x .and. y?=w664:bool)
                                n514 = case shown="False" w665 {
                                tunnel: w672 -> [_ _]
                                tunnel: w668 -> [_ _]
                                frame False {
                                }
                                frame True {
                                }
                                }
                                n515 = case shown="True" w664 {
                                tunnel: w667 -> [_ w674]
                                frame False {
                                n516 = local write "Temperature Control 4"(FALSE ("Temperature Control 4")) -> ()
                                }
                                frame True {
                                n517 = local write "Temperature SP 4"(w674) -> ()
                                n518 = local write "Temperature Control 4"(TRUE ("Temperature Control 5")) -> ()
                                }
                                }
                              }
                              frame #4 {
                                # "Bay 5"
                                n519 = Index Array(array=w688, index=5) -> (element=w686:dbl)
                                n520 = Index Array(array=w688, index=4) -> (element=w687:dbl)
                                n521 = script code="MATLAB script"("T5_SP"=w687, "P6"=w686) -> ()  [unwired: 1 in, 1 out]
                                n522 = Not Equal To 0?(x=w686) -> (x != 0?=w684:bool)
                                n523 = And(x=w684, y=w682) -> (x .and. y?=w683:bool)
                                n524 = local read "BAY 5"() -> (w677:u16)
                                n525 = Less Or Equal?(x=w677, y=u16 4) -> (x <= y?=w681:bool)
                                n526 = Greater Or Equal?(x=w677, y=u16 1) -> (x >= y?=w678:bool)
                                n527 = case shown="False" w683 {
                                tunnel: w691 -> [_ _]
                                tunnel: w686 -> [_ _]
                                frame False {
                                }
                                frame True {
                                }
                                }
                                n528 = And(x=w678, y=w681) -> (x .and. y?=w676:bool)
                                n529 = And(x=w676, y=w682) -> (x .and. y?=w685:bool)
                                n530 = case shown="True" w685 {
                                tunnel: w687 -> [_ w693]
                                frame False {
                                n531 = local write "Temperature Control 5"(FALSE ("Temperature Control 5")) -> ()
                                }
                                frame True {
                                n532 = local write "Temperature SP 5"(w693) -> ()
                                n533 = local write "Temperature Control 5"(TRUE ("Temperature Control 5")) -> ()
                                }
                                }
                              }
                            }
                          }
                          frame #1 {
                            # "Wait till Steady State temperature readings on all bays"
                            n534 = while {
                              tunnel: w696 -> [w697]
                              stop <- w698 stop-if-true
                              n535 = flat-sequence {
                                tunnel: [w701] -> w698
                                tunnel: w697 -> [w700]
                                frame #0 {
                                n536 = Wait (ms)(milliseconds to wait=u32 1500) -> ()  [unwired: 1 out]
                                }
                                frame #1 {
                                n537 = local read "Temp SS? 2"() -> (w704:bool)
                                n538 = local read "Temp SS? 3"() -> (w705:bool)
                                n539 = local read "Temp SS? 4"() -> (w706:bool)
                                n540 = local read "Temp SS? 5"() -> (w707:bool)
                                n541 = local read "Temp SS? 1"() -> (w703:bool)
                                n542 = Not(x=w700) -> (.not. x?=w713:bool)
                                n543 = local read "Stop"() -> (w702:bool)
                                n544 = And(x=w705, y=w706) -> (x .and. y?=w709:bool)
                                n545 = And(x=w703, y=w704) -> (x .and. y?=w710:bool)
                                n546 = And(x=w710, y=w709) -> (x .and. y?=w708:bool)
                                n547 = And(x=w708, y=w707) -> (x .and. y?=w711:bool)
                                n548 = Or(x=w713, y=w711) -> (x .or. y?=w712:bool)
                                n549 = Or(x=w712, y=w702) -> (x .or. y?=w701:bool)
                                }
                              }
                            }
                            n550 = local write "Calculate condition"(TRUE ("Calculate condition")) -> ()
                          }
                          frame #2 {
                            n551 = flat-sequence {
                              tunnel: w716 -> [w718]
                              tunnel: [w718] -> w715
                              tunnel: w715 -> [w723]
                              tunnel: [w723] -> w714
                              frame #0 {
                                n552 = local write "Equlibrating Temperature"(TRUE) -> ()
                              }
                              frame #1 {
                                # "Wait 1.5 system volumes"
                                n553 = local read "Number of System Flushes per condtion"() -> (w719:dbl)
                                n554 = local read "Extra system dead volume"() -> (w721:dbl)
                                n555 = script code="start = tic;\nP_tot = P1+P2+P3+P4+P5+P6;\nif P_tot >0\n  extra_res = extr_sys_dead_vol/P_tot;\nelse\n   extra_res =0;\nend\ntotal_sys_res = tau1 + tau2 + tau3 + tau4 + tau5 + extra_res;\ntotal_wait_time = total_sys_res*num_flush_per_cond*60;"("extr_sys_dead_vol"=w721, "num_flush_per_cond"=w719) -> ("??"=w724:errorcluster, "total_wait_time"=→"total_flush_time":dbl, "total_sys_res"=→"Total System Resisdence Time(min)":dbl)  [unwired: 1 in]
                                n556 = while {
                                tunnel: w723 -> [w726]
                                tunnel: w724 -> [w729]
                                stop <- w730 stop-if-true
                                # "Check if system is flushed every 10 seconds"
                                n557 = script code="end1 = toc(start);\nflush_time = 0;\ntotal_wait_time = 10;\nif end1 > total_wait_time\n   flush_time = 1;\nend\ncurr_wait_time = end1 /60;"("??"=w729) -> ("flush_time"=w733:dbl, "curr_wait_time"=w728:dbl)  [unwired: 1 out]
                                "curr_wait_time" <- w728
                                n558 = Not Equal To 0?(x=w733) -> (x != 0?=w732:bool)
                                n559 = Multiply(x=60.0, y=w728) -> ()  [unwired: 1 out]
                                n560 = local read "Stop"() -> (w735:bool)
                                n561 = Or(x=w732, y=w735) -> (x .or. y?=w731:bool)
                                n562 = Not(x=w726) -> (.not. x?=w725:bool)
                                n563 = Wait (ms)(milliseconds to wait=u32 10000) -> ()  [unwired: 1 out]
                                n564 = Or(x=w731, y=w725) -> (x .or. y?=w730:bool)
                                }
                              }
                            }
                          }
                          frame #3 {
                            # "Collect HPLC Data"
                            n565 = flat-sequence {
                              tunnel: w737 -> [w744]
                              tunnel: w736 -> [w743]
                              frame #0 {
                                n566 = local read "pause for ms"() -> (w740:bool)
                                n567 = case shown="True" w740 {
                                frame False {
                                }
                                frame True {
                                n568 = One Button Dialog(message="Press OK to Analyze Data", button name ("OK")="OK" ("Left Button Text (\"Yes\")")) -> ()  [unwired: 1 out]
                                }
                                }
                                n569 = local write "Flushing System"(TRUE ("Flushing System")) -> ()
                                "System Flushed?" <- TRUE ("System Flushed?")
                              }
                              frame #1 {
                                n570 = flat-sequence {
                                tunnel: [w746] -> w745
                                tunnel: w745 -> [w752]
                                tunnel: w744 -> [w760]
                                tunnel: w743 -> [w761]
                                frame #0 {
                                n571 = disable-structure shown="Enabled" {
                                disable-tunnel: [w747 _] -> w746
                                frame Disabled {
                                n572 = local read "COMM Port :: Milligat Pumps"() -> (w748:refnum<visa-resource-name>)
                                n573 = local read "P_tot"() -> (w751:dbl)
                                n574 = Multiply(x=w751, y=2.0) -> (x*y=w747:dbl)
                                n575 = call "PumpDispense.vi"("Flowrate(ul/min)"=w747, "Pump Address"="f", "Pump COMM Port"=w748) -> ()  [unwired: 7 in, 2 out]
                                }
                                frame Enabled {
                                }
                                }
                                }
                                frame #1 {
                                n576 = disable-structure shown="Enabled" {
                                disable-tunnel: w752 -> [w754 _]
                                frame Disabled {
                                n577 = local read "Stop"() -> (w753:bool)
                                n578 = case shown="False" w753 {
                                tunnel: w754 -> [w755 _]
                                frame False {
                                n579 = Divide(x=400.0 ("y"), y=w755) -> (x/y=w757:dbl)
                                n580 = Multiply(x=60000.0, y=w757) -> (x*y=w759:dbl)
                                n581 = Wait (ms)(milliseconds to wait=w759) -> ()  [unwired: 1 out]
                                }
                                frame True {
                                }
                                }
                                }
                                frame Enabled {
                                }
                                }
                                }
                                frame #2 {
                                n582 = while {
                                tunnel: w760 -> [w772]
                                tunnel: w761 -> [w766]
                                tunnel: w760 -> [w764]
                                stop <- w767 stop-if-true
                                n583 = flat-sequence {
                                tunnel: w764 -> [w773]
                                tunnel: w772 -> [_]
                                tunnel: [w828] -> w763
                                tunnel: [w827] -> w762
                                tunnel: w763 -> [w852]
                                tunnel: w762 -> [w851]
                                tunnel: [w871] -> w765
                                tunnel: [w873] -> w770
                                tunnel: w765 -> [w873]
                                frame #0 {
                                n584 = local read "COMM Port :: Milligat Pumps"() -> (w775:refnum<visa-resource-name>)
                                n585 = stacked-sequence {
                                tunnel: w775 -> [w778 w787 w796 w798 w804 w814]
                                tunnel: w773 -> [w777 w783 w793 w800 w806 w810]
                                tunnel: 1.0 ("Flowrate(ul/min)") -> [w776 w782 w791 w797 w803 w809]
                                frame #0 {
                                n586 = Index Array(array=w777, index=0) -> (element=w780:dbl)
                                n587 = Greater Than 0?(x=w780) -> (x > 0?=w779:bool)
                                n588 = case shown="True" w779 {
                                tunnel: w778 -> [_ _]
                                tunnel: w776 -> [_ _]
                                frame False {
                                }
                                frame True {
                                }
                                }
                                }
                                frame #1 {
                                n589 = Index Array(array=w783, index=1) -> (element=w785:dbl)
                                n590 = Greater Than 0?(x=w785) -> (x > 0?=w784:bool)
                                n591 = case shown="True" w784 {
                                tunnel: w782 -> [_ w789]
                                tunnel: w787 -> [_ w788]
                                frame False {
                                }
                                frame True {
                                n592 = local read "Syringe_pump?"() -> (w790:bool)
                                n593 = case shown="True" w790 {
                                tunnel: w789 -> [_ _]
                                tunnel: w788 -> [_ _]
                                frame False {
                                }
                                frame True {
                                n594 = disable-structure shown="Disabled" {
                                frame Disabled {
                                (unwired) u16 0 items=["Infuse", "Withdraw"] ("Run Direction (0:Infuse)")
                                (unwired) u32 4 items=["milliliters per hour (ml/hr)", "milliliters per minute (ml/min)", "milliliters per second (ml/sec)", "microliters per hour (ul/hr)", "microliters per minute (ul/min)", "microliters per second (ul/sec)", "nanoliters per hour (nl/hr)", "nanoliters per minute (nl/min)", "nanoliters per second (nl/sec)", "picoliters per hour (pl/hr)", "picoliters per minute (pl/min)", "picoliters per second (pl/sec)"] ("Flow Rate Units (1:ml/min)")
                                (unwired) u16 0 items=["Infuse", "Withdraw"] ("Pump Direction (0:Infuse)")
                                (unwired) i8 2 ("Pump Address")
                                n595 = local read "COMM Port:: Harvard Syringe Pump"() -> ()  [unwired: 1 out]
                                }
                                frame Enabled {
                                }
                                }
                                }
                                }
                                }
                                }
                                }
                                frame #2 {
                                n596 = Index Array(array=w793, index=2) -> (element=w794:dbl)
                                n597 = Greater Than 0?(x=w794) -> (x > 0?=w792:bool)
                                n598 = case shown="True" w792 {
                                tunnel: w796 -> [_ _]
                                tunnel: w791 -> [_ _]
                                frame False {
                                }
                                frame True {
                                }
                                }
                                }
                                frame #3 {
                                n599 = Index Array(array=w800, index=3) -> (element=w801:dbl)
                                n600 = Greater Than 0?(x=w801) -> (x > 0?=w799:bool)
                                n601 = case shown="True" w799 {
                                tunnel: w798 -> [_ _]
                                tunnel: w797 -> [_ _]
                                frame False {
                                }
                                frame True {
                                }
                                }
                                }
                                frame #4 {
                                n602 = Index Array(array=w806, index=4) -> (element=w807:dbl)
                                n603 = Greater Than 0?(x=w807) -> (x > 0?=w805:bool)
                                n604 = case shown="True" w805 {
                                tunnel: w804 -> [_ _]
                                tunnel: w803 -> [_ _]
                                frame False {
                                }
                                frame True {
                                }
                                }
                                }
                                frame #5 {
                                n605 = Index Array(array=w810, index=5) -> (element=w812:dbl)
                                n606 = Greater Than 0?(x=w812) -> (x > 0?=w811:bool)
                                n607 = case shown="True" w811 {
                                tunnel: w814 -> [_ _]
                                tunnel: w809 -> [_ _]
                                frame False {
                                }
                                frame True {
                                }
                                }
                                }
                                }
                                }
                                frame #1 {
                                n608 = while {
                                stop <- w820 stop-if-true
                                n609 = local read "Phase_Sensor_voltage"() -> (w815:dbl)
                                n610 = script code="organic_phase = 0;\nif start_phase_time \n   start_phase_timer = tic;\n   start_phase_time = 0;\nelse\n  %ignore phase sensor values\n  %if not(phase_sensor_val >2.9 && phase_sensor_val <3.8)\n    %    start_phase_timer = tic;\n   %end\n\n   end_phase_time =  toc(start_phase_timer )\n\n   if end_phase_time > 2\n       organic_phase = 1;\n       start_phase_time = 1;\n   end\n\nend"("phase_sensor_val"=w815) -> ("organic_phase"=w817:dbl)  [unwired: 1 in, 1 out]
                                n611 = local read "Stop"() -> (w819:bool)
                                n612 = Not Equal To 0?(x=w817) -> (x != 0?=w818:bool)
                                n613 = Or(x=w818, y=w819) -> (x .or. y?=w820:bool)
                                n614 = Wait (ms)(milliseconds to wait=u32 300) -> ()  [unwired: 1 out]
                                }
                                }
                                frame #2 {
                                n615 = local read "Stop"() -> (w822:bool)
                                n616 = Not(x=w822) -> (.not. x?=w821:bool)
                                n617 = local read "Sample Valve COMM::Port"() -> (w823:refnum<visa-resource-name>)
                                n618 = case shown="True" w821 {
                                tunnel: w823 -> [_ w824]
                                frame False {
                                }
                                frame True {
                                n619 = flat-sequence {
                                tunnel: w824 -> [_]
                                frame #0 {
                                (unwired) u8 22 ("DO Channel")
                                (unwired) FALSE ("Output Value")
                                (unwired) u8 22 ("DO Channel")
                                (unwired) TRUE ("Output Value")
                                n620 = disable-structure shown="Disabled" {
                                frame Disabled {
                                n621 = local read "Sample Valve COMM::Port"() -> ()  [unwired: 1 out]
                                }
                                frame Enabled {
                                }
                                }
                                n622 = flat-sequence {
                                frame #0 {
                                n623 = Wait (ms)(milliseconds to wait=u32 500) -> ()  [unwired: 1 out]
                                }
                                }
                                }
                                frame #1 {
                                n624 = Wait (ms)(milliseconds to wait=u32 2000) -> ()  [unwired: 1 out]
                                }
                                frame #2 {
                                }
                                }
                                }
                                }
                                }
                                frame #3 {
                                n625 = local read "Stop"() -> (w831:bool)
                                n626 = local read "Bay Parameters"() -> (w827:T2)
                                n627 = Unbundle By Name(w827) -> ("Hplc Wait time(min)"=w829:dbl)
                                n628 = Not(x=w831) -> (.not. x?=w830:bool)
                                n629 = case shown="True" w830 {
                                tunnel: w829 -> [_ w835]
                                tunnel: [errorcluster {"status"=FALSE, "code"=0, "source"=""} ("error out") w834] -> w828
                                tunnel: w827 -> [_ w833]
                                frame False {
                                }
                                frame True {
                                n630 = flat-sequence {
                                tunnel: w835 -> [w837]
                                tunnel: [w849] -> w834
                                tunnel: w833 -> [w848]
                                frame #0 {
                                # "Wait till for HPLC Method"
                                n631 = script code="start = tic;"() -> ("??"=w836:errorcluster)  [unwired: 1 in]
                                n632 = while {
                                tunnel: w837 -> [w839]
                                tunnel: w836 -> [w838]
                                stop <- w845 stop-if-true
                                n633 = Multiply(x=w839, y=60.0) -> (x*y=w840:dbl)
                                n634 = script code="end1 = toc(start);\nflush_time = 0;\nhplc_wait_time = 10;\nif end1 > hplc_wait_time\n   flush_time = 1;\nend"("??"=w838, "hplc_wait_time"=w840) -> ("flush_time"=w842:dbl)  [unwired: 1 out]
                                n635 = local read "Stop"() -> (w844:bool)
                                n636 = Not Equal To 0?(x=w842) -> (x != 0?=w843:bool)
                                n637 = Or(x=w843, y=w844) -> (x .or. y?=w845:bool)
                                }
                                }
                                frame #1 {
                                (unwired) u8 24 ("DO Channel")
                                (unwired) FALSE ("Output Value")
                                (unwired) u8 24 ("DO Channel")
                                (unwired) TRUE ("Output Value")
                                n638 = flat-sequence {
                                frame #0 {
                                n639 = Wait (ms)(milliseconds to wait=u32 500) -> ()  [unwired: 1 out]
                                }
                                }
                                }
                                frame #2 {
                                n640 = Wait (ms)(milliseconds to wait=u32 30000) -> ()  [unwired: 1 out]
                                }
                                frame #3 {
                                n641 = Unbundle By Name(w848) -> ("hplc File Name"=w850:string)
                                n642 = call "hplc_analyze.vi"("File Path"=w850) -> ("error out"=w849:errorcluster)  [unwired: 10 in]
                                }
                                }
                                }
                                }
                                }
                                frame #4 {
                                n643 = Unbundle By Name(w852) -> ("status"=w853:bool)
                                n644 = case shown="True" w853 {
                                tunnel: w851 -> [_ w854]
                                frame False {
                                }
                                frame True {
                                n645 = while {
                                tunnel: w854 -> [w856]
                                stop <- w855 stop-if-true
                                w861 = "An error occured while trying to read HPLC data. " ("message")
                                n646 = local write "Error Message"(w861) -> ()
                                n647 = call <vilib>:"Three Button Dialog.vi"("Right Button Text (\"Cancel\")"="STOP EXPs" ("F button name (\"Cancel\")"), "Center Button Text (\"No\")"="REDO" ("T button name (\"OK\")"), "Left Button Text (\"Yes\")"="REREAD" ("T button name (\"OK\")"), "message"=w861) -> ("Which Button?"=w857:T12)  [unwired: 7 in]
                                n648 = case shown="\"Right Button\"" w857 {
                                tunnel: w856 -> [_ _ w868 _]
                                tunnel: [TRUE TRUE w867 w870] -> w855
                                frame "Right Button" {
                                w862 = TRUE ("Setup Error")
                                n649 = local write "System Error"(w862) -> ()
                                n650 = local write "Setup Error"(w862) -> ()
                                n651 = script code="system_error = 1"() -> ()  [unwired: 1 in, 1 out]
                                n652 = local write "Stop"(w862) -> ()
                                }
                                frame "Center Button" {
                                n653 = script code="redo = true;\nopt_ctr = 1;\nCurrExp = CurrExp + 1;\nncall0 = ncall0 +1;\nif req_ctr == req_tot\n       opt_ctr = 3;\n  else\n     req_ctr = req_ctr +1;\nend"() -> ()  [unwired: 1 in, 1 out]
                                }
                                frame "Left Button" {
                                n654 = Unbundle By Name(w868) -> ("hplc File Name"=w869:string)
                                n655 = call "hplc_analyze.vi"("File Path"=w869) -> ("error out"=w865:errorcluster)  [unwired: 10 in]
                                n656 = Unbundle By Name(w865) -> ("status"=w866:bool)
                                n657 = Not(x=w866) -> (.not. x?=w867:bool)
                                }
                                frame "Window Close" {
                                w870 = TRUE
                                n658 = local write "Setup Error"(w870) -> ()
                                n659 = script code="system_error = 1"() -> ()  [unwired: 1 in, 1 out]
                                n660 = local write "Stop"(w870) -> ()
                                }
                                }
                                }
                                }
                                }
                                }
                                frame #5 {
                                n661 = script code="repeat = 0"() -> ("repeat"=w872:dbl)  [unwired: 1 in, 1 out]
                                n662 = Equal To 0?(x=w872) -> (x = 0?=w871:bool)
                                n663 = case shown="False" w871 {
                                frame False {
                                (unwired) 30.0 ("Flowrate(ul/min)")
                                (unwired) "f" ("Pump Address")
                                n664 = disable-structure shown="Disabled" {
                                frame Disabled {
                                n665 = local read "COMM Port :: Milligat Pumps"() -> ()  [unwired: 1 out]
                                }
                                frame Enabled {
                                }
                                }
                                }
                                frame True {
                                }
                                }
                                }
                                frame #6 {
                                n666 = disable-structure shown="Disabled" {
                                frame Disabled {
                                (unwired) u8 22 ("DO Channel")
                                (unwired) FALSE ("Output Value")
                                (unwired) u8 22 ("DO Channel")
                                (unwired) TRUE ("Output Value")
                                n667 = flat-sequence {
                                frame #0 {
                                n668 = Wait (ms)(milliseconds to wait=u32 500) -> ()  [unwired: 1 out]
                                }
                                }
                                }
                                frame Enabled {
                                }
                                }
                                }
                                }
                                n669 = local read "Stop"() -> (w771:bool)
                                n670 = Not(x=w766) -> (.not. x?=w769:bool)
                                n671 = Or(x=w771, y=w770) -> (x .or. y?=w768:bool)
                                n672 = Or(x=w768, y=w769) -> (x .or. y?=w767:bool)
                                }
                                }
                                }
                              }
                              frame #2 {
                                n673 = script code="C_measured =Conc;\nFvalues(end +1,:) = [Conc];"() -> ()  [unwired: 1 in, 1 out]
                                n674 = local write "HPLC Analysis"(TRUE ("HPLC Analysis")) -> ()
                              }
                            }
                          }
                          frame #4 {
                            n675 = local read "Stop"() -> (w877:bool)
                            n676 = Not(x=w877) -> (.not. x?=w876:bool)
                            n677 = case shown="True" w876 {
                              tunnel: [1.0 w888] -> w878
                              frame False {
                              }
                              frame True {
                                # "Save data to excel file"
                                n678 = local read "Bay Parameters"() -> (w886:T2)
                                n679 = Unbundle By Name(w886) -> ("Total Number of Experiments 2"=w885:dbl)
                                n680 = script code="analyze_labview_results"("ncall"=w885) -> ("terminate"=w888:dbl, "ncall0"=w887:dbl, "experiment_history"=w883:dbl[][], "Pbest"=w881:dbl[], "Tbest"=w882:dbl[], "best_exp_num"=w880:dbl)  [unwired: 1 in, 1 out]
                                n681 = local write "Flowrates(ul/min)_best"(w881) -> ()
                                n682 = local write "temperature_best"(w882) -> ()
                                n683 = local write "best_exp_num"(w880) -> ()
                                n684 = local write "Current Experiment"(w887) -> ()
                                n685 = local write "Total Number of Experiments"(w885) -> ()
                                n686 = call-poly <vilib>:"Array To Matrix.vi"("Real 2D Array"=w883) -> ("Real Matrix"=w884:T13)
                                n687 = local write "experiment history"(w884) -> ()
                              }
                            }
                          }
                          frame #5 {
                            n688 = local read "Num_exp_till_pause"() -> (w890:i32)
                            n689 = Increment(x=w890) -> (x+1=w889:i32)
                            n690 = local write "Num_exp_till_pause"(w889) -> ()
                          }
                          frame #6 {
                            # "Pause System"
                            n691 = local read "Bay Parameters"() -> (w898:T2)
                            n692 = Unbundle By Name(w898) -> ("Num_conditons_per_wait"=w897:dbl)
                            n693 = local read "Num_exp_till_pause"() -> (w896:i32)
                            n694 = Equal?(x=w897, y=w896) -> (x = y?=w895:bool)
                            n695 = local read "Run_Stop_cluster"() -> (w892:T7)
                            n696 = Unbundle By Name(w892) -> ("Stop Run Button"=w894:bool)
                            n697 = Or(x=w894, y=w895) -> (x .or. y?=w893:bool)
                            n698 = case shown="True" w893 {
                              tunnel: w897 -> [w901 _]
                              tunnel: w896 -> [w902 _]
                              tunnel: w892 -> [_ w904]
                              frame False {
                                n699 = Greater?(x=w902, y=w901) -> (0:w900:bool)
                                n700 = case shown="True" w900 {
                                frame False {
                                }
                                frame True {
                                n701 = local write "Num_exp_till_pause"(0 ("Num_exp_till_pause")) -> ()
                                }
                                }
                              }
                              frame True {
                                n702 = flat-sequence {
                                tunnel: w904 -> [w929]
                                frame #0 {
                                w908 = string[] ["e", "f", "g", "h", "i", "j"]
                                # "Turn off pumps and stop controling temperature"
                                n703 = stacked-sequence {
                                frame #0 {
                                n704 = local write "Temperature Control 1"(FALSE ("Temperature Control 1")) -> ()
                                }
                                frame #1 {
                                n705 = local write "Temperature Control 2"(FALSE ("Temperature Control 2")) -> ()
                                }
                                frame #2 {
                                n706 = local write "Temperature Control 3"(FALSE ("Temperature Control 3")) -> ()
                                }
                                frame #3 {
                                n707 = local write "Temperature Control 4"(FALSE ("Temperature Control 4")) -> ()
                                }
                                frame #4 {
                                n708 = local write "Temperature Control 5"(FALSE ("Temperature Control 5")) -> ()
                                }
                                }
                                n709 = local read "COMM Port:: Harvard Syringe Pump"() -> (w906:refnum<visa-resource-name>)
                                n710 = local read "Syringe_pump?"() -> (w905:bool)
                                n711 = local read "COMM Port :: Milligat Pumps"() -> (w907:refnum<visa-resource-name>)
                                n712 = Array Size(array=w908) -> (size(s)=w909:i32)
                                n713 = case shown="True" w905 {
                                tunnel: w906 -> [_ _]
                                frame False {
                                }
                                frame True {
                                }
                                }
                                n714 = for {
                                N: w909 -> [_]
                                tunnel: w908 -> [_] mode=indexing
                                tunnel: w907 -> [_]
                                }
                                }
                                frame #1 {
                                n715 = local read "Stop"() -> (w917:bool)
                                n716 = Not(x=w917) -> (.not. x?=w916:bool)
                                n717 = case shown="True" w916 {
                                frame False {
                                }
                                frame True {
                                n718 = while {
                                stop <- w923 stop-if-true
                                # "Wait till user confirms system resume"
                                n719 = Two Button Dialog(message="System is currently paused. Refill Syringes, flush lines, then press OK to continue optimization.\nOr Redo to repeat condition ", 1:"REDO" ("F button name (\"Cancel\")"), 2:"OK" ("Left Button Text (\"Yes\")")) -> (T button?=w919:bool)
                                n720 = case shown="False" w919 {
                                tunnel: [TRUE TRUE] -> w918
                                frame False {
                                n721 = script code="redo = true;"() -> ()  [unwired: 1 in, 1 out]
                                }
                                frame True {
                                }
                                }
                                n722 = local read "Stop"() -> (w924:bool)
                                n723 = Or(x=w918, y=w924) -> (x .or. y?=w923:bool)
                                }
                                }
                                }
                                n724 = local write "stop_xl_write"(TRUE ("stop_xl_write")) -> ()
                                }
                                frame #2 {
                                n725 = local write "Num_exp_till_pause"(0 ("Num_exp_till_pause")) -> ()
                                n726 = Bundle By Name(cluster=w929, "Stop Run Button"=FALSE) -> (w927:T7)
                                n727 = local write "Run_Stop_cluster"(w927) -> ()
                                }
                                }
                              }
                            }
                          }
                          frame #7 {
                            w932 = FALSE
                            n728 = local write "Equlibrating Temperature"(w932) -> ()
                            n729 = local write "Calculate condition"(w932) -> ()
                            n730 = local write "Flushing System"(w932) -> ()
                            n731 = local write "HPLC Analysis"(w932) -> ()
                            n732 = local write "stop_xl_write"(TRUE ("stop_xl_write")) -> ()
                          }
                        }
                        n733 = while {
                          stop <- w959 stop-if-true
                          n734 = flat-sequence {
                            frame #0 {
                              n735 = script code="save_excel_time_data;"() -> ()  [unwired: 1 in, 1 out]
                            }
                            frame #1 {
                              n736 = Wait (ms)(milliseconds to wait=u32 30000) -> ()  [unwired: 1 out]
                            }
                          }
                          n737 = local read "Stop"() -> (w960:bool)
                          n738 = local read "stop_xl_write"() -> (w958:bool)
                          n739 = Or(x=w958, y=w960) -> (x .or. y?=w959:bool)
                        }
                      }
                    }
                  }
                }
                n740 = Greater?(x=w534, y=w535) -> (0:w542:bool)
                n741 = Equal?(x=w540, y=1.0) -> (x = y?=w536:bool)
                n742 = local read "Stop"() -> (w543:bool)
                n743 = Or(x=w543, y=w542) -> (x .or. y?=w539:bool)
                n744 = Or(x=w536, y=w539) -> (x .or. y?=w538:bool)
                n745 = case shown="True" w536 {
                  frame False {
                  }
                  frame True {
                    w547 = u16 2 items=["System  Error", "System Running", "System Standby"] ("System Status")
                    n746 = local write "Stop"(TRUE ("Stop")) -> ()
                    n747 = local write "System Status"(w547) -> ()
                  }
                }
                "Optimization_loop_index" <- w544
              }
            }
          }
          n748 = while {
            stop <- w1050 stop-if-true
            n749 = local read "Temperature Control 3"() -> (w1046:bool)
            n750 = local read "Debug_run_button"() -> (w1047:bool)
            n751 = Not(x=w1047) -> (.not. x?=w1049:bool)
            n752 = And(x=w1049, y=w1046) -> (x .and. y?=w1048:bool)
            n753 = case shown="True" w1048 {
              frame False {
                n754 = local write "Temp SS? 3"(TRUE) -> ()
              }
              frame True {
                # "Bay 3 Temperature Controller"
                n755 = local read "Temperature SP 3"() -> (w1053:dbl)
                n756 = local read "Temperature 3"() -> (w1056:dbl)
                n757 = Subtract(x=w1056, y=w1053) -> (x-y=w1065:dbl)
                n758 = Absolute Value(x=w1065) -> (abs(x)=w1067:dbl)
                n759 = Less Or Equal?(x=w1067, y=1.2) -> (x <= y?=w1064:bool)
                n760 = local write "Temp SS? 3"(w1064) -> ()
                n761 = local read "SSR Duration 3"() -> (w1074:dbl)
                n762 = call-poly <vilib>:"PID Online Autotuning.vi"("setpoint"=w1053, "manipulated variable"=w1074, "autotuning parameters"=T9 {"type of controller"=enum."PID", "relay cycles"=3, "relay amplitude"=1.0, "control specifications"=enum."Normal", "PV noise level"=0.1} ("Autotuning Parameters R1"), "process variable"=w1056, "PID gains in"=T8 {"Proportional gain Kc"=0.38538, "Integral time Ti (sec)"=0.524375, "Derivative time Ti (sec)"=0.12585} ("PID gains 2")) -> ("setpoint out"=w1072:dbl, "process variable out"=w1073:dbl, "PID gains out"=w1076:T11)  [unwired: 6 in, 2 out]
                n763 = Greater?(x=w1053, y=w1056) -> (0:w1063:bool)
                n764 = call <vilib>:"PID Autotuning (Temperature).vi"("desired temperature"=w1072, "measured temperature"=w1073, "PID gains in"=w1076, "output range"=cluster{"output high":dbl, "output low":dbl} {"output high"=3.0, "output low"=-1.0} ("Output range")) -> ("output"=w1069:dbl)  [unwired: 12 in, 3 out]
                n765 = Multiply(x=1000.0, y=w1069) -> (x*y=w1071:dbl)
                n766 = local write "SSR Duration 3"(w1069) -> ()
                n767 = Greater Than 0?(x=w1071) -> (x > 0?=w1062:bool)
                n768 = And(x=w1062, y=w1063) -> (x .and. y?=w1060:bool)
                n769 = Subtract(x=w1056, y=10.0) -> (x-y=w1058:dbl)
                n770 = Less?(x=w1058, y=w1053) -> (x < y?=w1061:bool)
                n771 = And(x=w1061, y=w1060) -> (x .and. y?=w1059:bool)
                n772 = case shown="False" w1059 {
                  tunnel: [errorcluster {"status"=FALSE, "code"=0, "source"=""} ("error out") errorcluster {"status"=FALSE, "code"=0, "source"=""} ("error out")] -> _
                  tunnel: 4 -> [_ _]
                  tunnel: w1071 -> [w1082 _]
                  tunnel: [0.0 w1087] -> w1054
                  tunnel: w1053 -> [_ w1086]
                  frame False {
                    n773 = Absolute Value(x=w1082) -> (abs(x)=w1083:dbl)
                    n774 = Wait (ms)(milliseconds to wait=w1083) -> ()  [unwired: 1 out]
                  }
                  frame True {
                    n775 = script code="tempdiff3= SP3 - T3;\nif tempdiff3 > 10\n  if slope3 < .01\n     temp_check3 = temp_check3 + 1;\n  else\n      temp_check3 =0;\n  end\nend\n\nif temp_check3 > 9\n  temp_error3 = 1\nend"("SP3"=w1086) -> ("temp_error3"=w1087:dbl)  [unwired: 1 in, 1 out]
                  }
                }
                n776 = Not Equal To 0?(x=w1054) -> (x != 0?=w1055:bool)
                n777 = case shown="True" w1055 {
                  frame False {
                  }
                  frame True {
                    n778 = local write "Error Message"("Bay 3 Temperature Heating Error") -> ()
                  }
                }
                n779 = case shown="True" w1055 {
                  tunnel: w1055 -> [_ w1080]
                  frame False {
                  }
                  frame True {
                    n780 = local write "System Error"(w1080) -> ()
                    n781 = local write "Stop"(w1080) -> ()
                  }
                }
              }
            }
            n782 = Wait (ms)(milliseconds to wait=u32 400) -> ()  [unwired: 1 out]
            n783 = local read "Stop"() -> (w1050:bool)
          }
          n784 = while {
            stop <- w1008 stop-if-true
            n785 = local read "Debug_run_button"() -> (w1004:bool)
            n786 = Not(x=w1004) -> (.not. x?=w1007:bool)
            n787 = Wait (ms)(milliseconds to wait=u32 400) -> ()  [unwired: 1 out]
            n788 = local read "Temperature Control 4"() -> (w1006:bool)
            n789 = And(x=w1007, y=w1006) -> (x .and. y?=w1005:bool)
            n790 = case shown="True" w1005 {
              frame False {
                n791 = local write "Temp SS? 4"(TRUE ("Temp SS? 4")) -> ()
              }
              frame True {
                # "Bay 4 Temperature Controller"
                n792 = local read "Temperature SP 4"() -> (w1013:dbl)
                n793 = local read "Temperature 4"() -> (w1016:dbl)
                n794 = Subtract(x=w1016, y=w1013) -> (x-y=w1023:dbl)
                n795 = Absolute Value(x=w1023) -> (abs(x)=w1025:dbl)
                n796 = Less Or Equal?(x=w1025, y=1.2) -> (x <= y?=w1022:bool)
                n797 = local write "Temp SS? 4"(w1022) -> ()
                n798 = local read "SSR Duration 4"() -> (w1026:dbl)
                n799 = call-poly <vilib>:"PID Online Autotuning.vi"("setpoint"=w1013, "manipulated variable"=w1026, "autotuning parameters"=T9 {"type of controller"=enum."PID", "relay cycles"=3, "relay amplitude"=1.0, "control specifications"=enum."Normal", "PV noise level"=0.1} ("Autotuning Parameters R1"), "process variable"=w1016, "PID gains in"=T8 {"Proportional gain Kc"=0.38538, "Integral time Ti (sec)"=0.524375, "Derivative time Ti (sec)"=0.12585} ("PID gains 2")) -> ("setpoint out"=w1028:dbl, "process variable out"=w1029:dbl, "PID gains out"=w1031:T11)  [unwired: 6 in, 2 out]
                n800 = call <vilib>:"PID Autotuning (Temperature).vi"("desired temperature"=w1028, "measured temperature"=w1029, "PID gains in"=w1031, "output range"=cluster{"output high":dbl, "output low":dbl} {"output high"=3.0, "output low"=-1.0} ("Output range")) -> ("output"=w1027:dbl)  [unwired: 12 in, 3 out]
                n801 = Subtract(x=w1016, y=10.0) -> (x-y=w1015:dbl)
                n802 = Less?(x=w1015, y=w1013) -> (x < y?=w1017:bool)
                n803 = Multiply(x=1000.0, y=w1027) -> (x*y=w1035:dbl)
                n804 = Greater?(x=w1013, y=w1016) -> (0:w1021:bool)
                n805 = Greater Than 0?(x=w1035) -> (x > 0?=w1020:bool)
                n806 = local write "SSR Duration 4"(w1027) -> ()
                n807 = And(x=w1020, y=w1021) -> (x .and. y?=w1019:bool)
                n808 = And(x=w1017, y=w1019) -> (x .and. y?=w1018:bool)
                n809 = case shown="False" w1018 {
                  tunnel: [errorcluster {"status"=FALSE, "code"=0, "source"=""} ("error out") errorcluster {"status"=FALSE, "code"=0, "source"=""} ("error out")] -> _
                  tunnel: 5 -> [_ _]
                  tunnel: w1035 -> [w1040 _]
                  tunnel: w1013 -> [_ w1045]
                  tunnel: [0.0 w1044] -> w1012
                  frame False {
                    n810 = Absolute Value(x=w1040) -> (abs(x)=w1041:dbl)
                    n811 = Wait (ms)(milliseconds to wait=w1041) -> ()  [unwired: 1 out]
                  }
                  frame True {
                    n812 = script code="tempdiff4= SP4 - T4;\nif tempdiff4 > 10\n  if slope4 < .01\n     temp_check4 = temp_check4 + 1;\n  else\n      temp_check4 =0;\n  end\nend\n\nif temp_check4 > 9\n  temp_error4 = 1\nend"("SP4"=w1045) -> ("temp_error4"=w1044:dbl)  [unwired: 1 in, 1 out]
                  }
                }
                n813 = Not Equal To 0?(x=w1012) -> (x != 0?=w1011:bool)
                n814 = case shown="True" w1011 {
                  frame False {
                  }
                  frame True {
                    n815 = local write "Error Message"("Bay 4 Temperature Heating Error") -> ()
                  }
                }
                n816 = case shown="True" w1011 {
                  tunnel: w1011 -> [_ w1038]
                  frame False {
                  }
                  frame True {
                    n817 = local write "System Error"(w1038) -> ()
                    n818 = local write "Stop"(w1038) -> ()
                  }
                }
              }
            }
            n819 = local read "Stop"() -> (w1008:bool)
          }
          n820 = while {
            stop <- w529 stop-if-true
            n821 = script code="TempArr1=circshift(TempArr1,9);\nTempArr2=circshift(TempArr2,9);\nTempArr3=circshift(TempArr3,9);\nTempArr4=circshift(TempArr4,9);\nTempArr5=circshift(TempArr5,9);\n\nTempArr1(10)=T1;\nTempArr2(10)=T2;\nTempArr3(10)=T3;\nTempArr4(10)=T4;\nTempArr5(10)=T5;\n\n[slope1 temp] = polyfit([1,2,3,4,5,6,7,8,9,10]',TempArr1,1);\nslope1 = slope1(1);\n[slope2 temp] = polyfit([1,2,3,4,5,6,7,8,9,10]',TempArr2,1);\nslope2= slope2(1);\n[slope3 temp] = polyfit([1,2,3,4,5,6,7,8,9,10]',TempArr3,1);\nslope3 = slope3(1);\n[slope4 temp] = polyfit([1,2,3,4,5,6,7,8,9,10]',TempArr4,1);\nslope4 = slope4(1);\n[slope5 temp] = polyfit([1,2,3,4,5,6,7,8,9,10]',TempArr5,1);\nslope5 = slope5(1);"() -> ()  [unwired: 1 in, 1 out]
            n822 = Wait (ms)(milliseconds to wait=u32 600) -> ()  [unwired: 1 out]
            n823 = local read "Stop"() -> (w529:bool)
          }
          n824 = while {
            stop <- w966 stop-if-true
            n825 = local read "Debug_run_button"() -> (w963:bool)
            n826 = Not(x=w963) -> (.not. x?=w965:bool)
            n827 = local read "Temperature Control 5"() -> (w962:bool)
            n828 = And(x=w965, y=w962) -> (x .and. y?=w964:bool)
            n829 = case shown="True" w964 {
              frame False {
                n830 = local write "Temp SS? 5"(TRUE ("Temp SS? 5")) -> ()
              }
              frame True {
                # "Bay 5 Temperature Controller"
                n831 = local read "SSR Duration 5"() -> (w984:dbl)
                n832 = local read "Temperature SP 5"() -> (w970:dbl)
                n833 = local read "Temperature 5"() -> (w973:dbl)
                n834 = Subtract(x=w973, y=w970) -> (x-y=w981:dbl)
                n835 = Absolute Value(x=w981) -> (abs(x)=w983:dbl)
                n836 = Less Or Equal?(x=w983, y=1.2) -> (x <= y?=w980:bool)
                n837 = local write "Temp SS? 5"(w980) -> ()
                n838 = call-poly <vilib>:"PID Online Autotuning.vi"("setpoint"=w970, "manipulated variable"=w984, "autotuning parameters"=T9 {"type of controller"=enum."PID", "relay cycles"=3, "relay amplitude"=1.0, "control specifications"=enum."Normal", "PV noise level"=0.1} ("Autotuning Parameters R1"), "process variable"=w973, "PID gains in"=T8 {"Proportional gain Kc"=0.38538, "Integral time Ti (sec)"=0.524375, "Derivative time Ti (sec)"=0.12585} ("PID gains 2")) -> ("setpoint out"=w986:dbl, "process variable out"=w987:dbl, "PID gains out"=w989:T11)  [unwired: 6 in, 2 out]
                n839 = call <vilib>:"PID Autotuning (Temperature).vi"("desired temperature"=w986, "measured temperature"=w987, "PID gains in"=w989, "output range"=cluster{"output high":dbl, "output low":dbl} {"output high"=3.0, "output low"=-1.0} ("Output range")) -> ("output"=w985:dbl)  [unwired: 12 in, 3 out]
                n840 = Multiply(x=1000.0, y=w985) -> (x*y=w993:dbl)
                n841 = Greater?(x=w970, y=w973) -> (0:w978:bool)
                n842 = Greater Than 0?(x=w993) -> (x > 0?=w979:bool)
                n843 = local write "SSR Duration 5"(w985) -> ()
                n844 = And(x=w979, y=w978) -> (x .and. y?=w976:bool)
                n845 = Subtract(x=w973, y=10.0) -> (x-y=w974:dbl)
                n846 = Greater?(x=w974, y=w970) -> (0:w977:bool)
                n847 = And(x=w977, y=w976) -> (x .and. y?=w975:bool)
                n848 = case shown="True" w975 {
                  tunnel: [errorcluster {"status"=FALSE, "code"=0, "source"=""} ("error out") errorcluster {"status"=FALSE, "code"=0, "source"=""} ("error out")] -> _
                  tunnel: 6 -> [_ _]
                  tunnel: w993 -> [w998 _]
                  tunnel: [0.0 w1003] -> w971
                  tunnel: w970 -> [_ w1002]
                  frame False {
                    n849 = Absolute Value(x=w998) -> (abs(x)=w999:dbl)
                    n850 = Wait (ms)(milliseconds to wait=w999) -> ()  [unwired: 1 out]
                  }
                  frame True {
                    n851 = script code="tempdiff5= SP5 - T5;\n\nif tempdiff5 > 10\n  if slope5 < .01\n     temp_check5 = temp_check5 + 1;\n  else\n      temp_check5 =0;\n  end\nend\n\nif temp_check5 >9\n  temp_error5 = 1\nend"("SP5"=w1002) -> ("temp_error5"=w1003:dbl)  [unwired: 1 in, 1 out]
                  }
                }
                n852 = Not Equal To 0?(x=w971) -> (x != 0?=w969:bool)
                n853 = case shown="True" w969 {
                  frame False {
                  }
                  frame True {
                    n854 = local write "Error Message"("Bay 5 Temperature Heating Error") -> ()
                  }
                }
                n855 = case shown="True" w969 {
                  tunnel: w969 -> [_ w996]
                  frame False {
                  }
                  frame True {
                    n856 = local write "Stop"(w996) -> ()
                    n857 = local write "System Error"(w996) -> ()
                  }
                }
              }
            }
            n858 = Wait (ms)(milliseconds to wait=u32 400) -> ()  [unwired: 1 out]
            n859 = local read "Stop"() -> (w966:bool)
          }
        }
      }
      n860 = while {
        tunnel: errorcluster {"status"=FALSE, "code"=0, "source"=""} ("error out") -> [w122]
        stop <- w137 stop-if-true
        w113 = FALSE
        # "Bay 5 Temperature Read"
        # "Bay 4 Temperature Read"
        # "Bay 3 Temperature Read"
        # "Bay 2 Temperature Read"
        # "Bay 1 Temperature Read"
        n861 = local read "Stop"() -> (w137:bool)
        n862 = local read "Temperature SP 1"() -> (w130:dbl)
        n863 = call-poly <vilib>:"PID Control Input Filter.vi"("input"=w130) -> ("output"=w128:dbl)  [unwired: 4 in]
        n864 = case shown="False" w113 {
          tunnel: w127 -> [w146 _]
          tunnel: [w146 w147] -> w134
          frame False {
            n865 = local write "Temperature 1"(w146) -> ()
          }
          frame True {
            n866 = local read "Temperature 1"() -> (w147:dbl)
          }
        }
        n867 = flat-sequence {
          tunnel: w128 -> [w156]
          tunnel: [w156] -> w127
          frame #0 {
            n868 = Wait (ms)(milliseconds to wait=u32 100) -> ()  [unwired: 1 out]
          }
        }
        n869 = local read "Temperature SP 2"() -> (w129:dbl)
        n870 = call-poly <vilib>:"PID Control Input Filter.vi"("input"=w129) -> ("output"=w126:dbl)  [unwired: 4 in]
        n871 = case shown="True" w113 {
          tunnel: w125 -> [w144 _]
          tunnel: [w144 w145] -> w133
          frame False {
            n872 = local write "Temperature 2"(w144) -> ()
          }
          frame True {
            n873 = local read "Temperature 2"() -> (w145:dbl)
          }
        }
        n874 = flat-sequence {
          tunnel: w126 -> [w154]
          tunnel: [w154] -> w125
          frame #0 {
            n875 = Wait (ms)(milliseconds to wait=u32 100) -> ()  [unwired: 1 out]
          }
        }
        n876 = local read "Temperature SP 3"() -> (w123:dbl)
        n877 = case shown="False" w113 {
          tunnel: w120 -> [w142 _]
          tunnel: [w142 w143] -> w124
          frame False {
            n878 = local write "Temperature 3"(w142) -> ()
          }
          frame True {
            n879 = local read "Temperature 3"() -> (w143:dbl)
          }
        }
        n880 = call-poly <vilib>:"PID Control Input Filter.vi"("input"=w123) -> ("output"=w121:dbl)  [unwired: 4 in]
        n881 = flat-sequence {
          tunnel: w121 -> [w152]
          tunnel: [w152] -> w120
          frame #0 {
            n882 = Wait (ms)(milliseconds to wait=u32 100) -> ()  [unwired: 1 out]
          }
        }
        n883 = local read "Temperature SP 4"() -> (w119:dbl)
        n884 = case shown="True" w113 {
          tunnel: w117 -> [w140 _]
          tunnel: [w140 w141] -> w132
          frame False {
            n885 = local write "Temperature 4"(w140) -> ()
          }
          frame True {
            n886 = local read "Temperature 4"() -> (w141:dbl)
          }
        }
        n887 = call-poly <vilib>:"PID Control Input Filter.vi"("input"=w119) -> ("output"=w118:dbl)  [unwired: 4 in]
        n888 = flat-sequence {
          tunnel: w118 -> [w150]
          tunnel: [w150] -> w117
          frame #0 {
            n889 = Wait (ms)(milliseconds to wait=u32 100) -> ()  [unwired: 1 out]
          }
        }
        n890 = local read "Temperature SP 5"() -> (w116:dbl)
        n891 = flat-sequence {
          tunnel: w115 -> [w148]
          tunnel: [w148] -> w114
          frame #0 {
            n892 = Wait (ms)(milliseconds to wait=u32 100) -> ()  [unwired: 1 out]
          }
        }
        n893 = call-poly <vilib>:"PID Control Input Filter.vi"("input"=w116) -> ("output"=w115:dbl)  [unwired: 4 in]
        n894 = local write "error out"(w122) -> ()
        n895 = Build Array(w134, w133, w124, w132, w114) -> (w136:dbl[])
        n896 = Array To Cluster(array=w136) -> (cluster=→"Teperature Chart":T5)
        n897 = case shown="False" w113 {
          tunnel: w114 -> [w138 _]
          tunnel: [w138 w139] -> w131
          frame False {
            n898 = local write "Temperature 5"(w138) -> ()
          }
          frame True {
            n899 = local read "Temperature 5"() -> (w139:dbl)
          }
        }
        n900 = script code="MATLAB script"("T1"=w134, "T2"=w133, "T3"=w124, "T4"=w132, "T5"=w131) -> ()  [unwired: 1 in, 1 out]
      }
      n901 = while {
        stop <- w78 stop-if-true
        n902 = local read "Pump setpoint(ul/min) 1"() -> (w81:dbl)
        n903 = local read "Pump setpoint(ul/min) 2"() -> (w77:dbl)
        n904 = local read "Pump setpoint(ul/min) 3"() -> (w76:dbl)
        n905 = local read "Pump setpoint(ul/min) 4"() -> (w75:dbl)
        n906 = local read "Pump setpoint(ul/min) 5"() -> (w74:dbl)
        n907 = local read "Pump setpoint(ul/min) 6"() -> (w73:dbl)
        n908 = Build Array(w81, w77, w76, w75, w74, w73) -> (w82:dbl[])
        n909 = Array To Cluster(array=w82) -> (cluster=→"Pump Setpoints Chart":T5)
        n910 = Wait (ms)(milliseconds to wait=u32 5000) -> ()  [unwired: 1 out]
        n911 = local read "Stop"() -> (w78:bool)
      }
      n912 = while {
        stop <- w62 stop-if-true
        n913 = local read "System Error"() -> (w61:bool)
        n914 = Wait (ms)(milliseconds to wait=u32 300) -> ()  [unwired: 1 out]
        n915 = case shown="True" w61 {
          tunnel: [w66 w67] -> w59
          frame False {
            w63 = u16 2 items=["System  Error", "System Running", "System Standby"] ("System Status")
            w64 = u16 1 items=["System  Error", "System Running", "System Standby"] ("System Status")
            n916 = local read "running?"() -> (w65:bool)
            n917 = Select(t=w64, s=w65, f=w63) -> (s? t:f=w66:u16)
          }
          frame True {
            w67 = u16 0 items=["System  Error", "System Running", "System Standby"] ("System Status")
          }
        }
        n918 = local read "Stop"() -> (w62:bool)
        n919 = local write "System Status"(w59) -> ()
      }
      n920 = while {
        stop <- w72 stop-if-true
        w68 = u8 0 ("Analog Channel")
        n921 = Wait (ms)(milliseconds to wait=u32 300) -> ()  [unwired: 1 out]
        n922 = Build Array(w68) -> (w69:u8[])
        n923 = Array To Cluster(array=w69) -> (cluster=→"Phase Sensor Chart":T3)
        n924 = local read "Stop"() -> (w72:bool)
        "Phase_Sensor_voltage" <- w68
      }
      n925 = while {
        stop <- w108 stop-if-true
        w90 = 270
        w84 = 600
        w85 = 600
        w83 = i32[] [1, 1, 14, 15]
        # "Read Pressure and Flowrate"
        n926 = local read "Stop"() -> (w108:bool)
        n927 = Index Array(array=w83, index=1) -> (element=w104:i32)
        n928 = Index Array(array=w83, index=0) -> (element=w105:i32)
        n929 = call-poly <vilib>:"PID Control Input Filter.vi"("input"=w104) -> ("output"=w97:dbl)  [unwired: 4 in]
        n930 = call-poly <vilib>:"PID Control Input Filter.vi"("input"=w105) -> ("output"=w96:dbl)  [unwired: 4 in]
        n931 = Multiply(x=104.96 ("y"), y=w97) -> (x*y=w98:dbl)
        n932 = Multiply(x=104.96 ("y"), y=w96) -> (x*y=w101:dbl)
        n933 = Subtract(x=w98, y=24.077) -> (x-y=w88:dbl)
        n934 = Subtract(x=w101, y=24.077) -> (x-y=w89:dbl)
        n935 = Build Array(w85, w84) -> (w93:i32[])
        n936 = Array To Cluster(array=w93) -> (cluster=→"Flowrate Chart":T4)
        n937 = Build Array(w89, w88) -> (w94:dbl[])
        n938 = local write "Flowrate Sensor 1"(w85) -> ()
        n939 = local write "Flowrate Sensor 2"(w84) -> ()
        n940 = local write "Pressure 1"(w89) -> ()
        n941 = local write "Pressure 2"(w88) -> ()
        n942 = Array To Cluster(array=w94) -> (cluster=→"Pressure Chart":T5)
        n943 = Wait (ms)(milliseconds to wait=u32 500) -> ()  [unwired: 1 out]
        n944 = script code="MATLAB script"("F1"=w85, "F2"=w84, "Pres1"=w89, "Pres2"=w88) -> ()  [unwired: 1 in, 1 out]
        n945 = Greater?(x=w88, y=w90) -> (0:w86:bool)
        n946 = Greater?(x=w89, y=w90) -> (0:w87:bool)
        n947 = case shown="True" w87 {
          frame False {
          }
          frame True {
            w112 = TRUE ("Stop")
            n948 = local write "System Error"(w112) -> ()
            n949 = local write "Stop"(w112) -> ()
            n950 = local write "Error Message"("Pressure Sensor 1 readings above 250psi") -> ()
            n951 = script code="system_error = 1;"() -> ()  [unwired: 1 in, 1 out]
          }
        }
        n952 = case shown="False" w86 {
          frame False {
          }
          frame True {
            w110 = TRUE ("Stop")
            n953 = local write "System Error"(w110) -> ()
            n954 = local write "Error Message"("Pressure Sensor 2 readings above 250psi") -> ()
            n955 = local write "Stop"(w110) -> ()
            n956 = script code="system_error = 1;"() -> ()  [unwired: 1 in, 1 out]
          }
        }
      }
    }
    frame #3 {
      # "Save and close xml and excel file"
      n957 = script code="if exist('xl_file','var') & exist('xlApp','var')\n  xlWorkbook.SaveAs(xl_file);\n  xlWorkbook.Close;\n  xlApp.Quit;\n  xlApp.delete;\nend"() -> ()  [unwired: 1 in, 1 out]
    }
    frame #4 {
      w1180 = string[] ["e", "f", "g", "h", "i", "j"]
      # "End communication to hardware"
      n958 = local read "Syringe_pump?"() -> (w1178:bool)
      n959 = local read "COMM Port:: Harvard Syringe Pump"() -> (w1179:refnum<visa-resource-name>)
      n960 = local read "COMM Port :: Milligat Pumps"() -> (w1182:refnum<visa-resource-name>)
      n961 = Array Size(array=w1180) -> (size(s)=w1181:i32)
      n962 = case shown="True" w1178 {
        tunnel: w1179 -> [_ _]
        frame False {
        }
        frame True {
        }
      }
      n963 = for {
        N: w1181 -> [_]
        tunnel: w1180 -> [_] mode=indexing
        tunnel: w1182 -> [_]
        n964 = Wait (ms)(milliseconds to wait=u32 100) -> ()  [unwired: 1 out]
      }
    }
    frame #5 {
      # "Display Error Messages if necessary"
      n965 = local read "Error Message"() -> (w1184:string)
      n966 = One Button Dialog(message=w1184) -> ()  [unwired: 1 in, 1 out]
    }
  }
